vi "main.vi"() -> ()   [LabVIEW 2020]
uses:
  <vilib>/Platform/TimedLoop/XDataNode/wakeup.ctl
  <vilib>/Platform/TimedLoop/XDataNode/XDNodeRunTimeDep.lvlib
  <vilib>/Platform/TimedLoop/XDataNode/nitl_modes.ctl
  <vilib>/Platform/TimedLoop/XDataNode/timing_clust.ctl
  <vilib>/Platform/TimedLoop/XDataNode/XDataNode.xnode
  <vilib>/addons/control/pid/NI_PID_pid.lvlib
  <vilib>/addons/control/pid/pid.llb/PID (DBL).vi
  <vilib>/imathl/engines/lvmath/Functions/Error Handling/Create Error.vi
  <vilib>/imath/engines/lvmath2/RunTimeEngine/BuiltInFunctions/diag/NIMS_diag.vi
  <vilib>/imath/engines/lvmath2/RunTimeEngine/NodeEndStatement/NIMS_NodeEndStatement_Output.vi
  <vilib>/imath/engines/lvmath2/RunTimeEngine/ErrorHandling/NIMS_Finalize Error.vi
  <vilib>/imath/engines/lvmath2/RunTimeEngine/IndexReplace/NIMS M($,S)=V.vi
  <vilib>/imath/engines/lvmath2/RunTimeEngine/IndexRead/NIMS V(S).vi
  <vilib>/imath/engines/lvmath2/RunTimeEngine/ErrorHandling/NIMS_Create Error From Enums.vi
  <vilib>/imath/engines/lvmath2/RunTimeEngine/RangeToken/NIMS_Range_R2 - Integer.vi
  <vilib>/imath/engines/lvmath2/RunTimeEngine/VariableToken/NIMS_VariableToken_CondDefinedDefinedByReplace.vi
  <vilib>/imath/engines/lvmath2/RunTimeEngine/IndexReplace/NIMS V(S)=S.vi
  <vilib>/imath/engines/lvmath2/RunTimeEngine/CommandStatement/MC_CommandStatement_break.vi
  <vilib>/imath/engines/lvmath2/RunTimeEngine/VariableToken/NIMS_VariableToken_CondDefined.vi
  <vilib>/imath/engines/lvmath2/RunTimeEngine/IndexRead/NIMS V($).vi
  <vilib>/imath/engines/lvmath2/RunTimeEngine/ArithmeticOperatorToken/NIMS_ArithmeticOperator_rightdiv(C,C).vi
  <vilib>/imath/engines/lvmath2/RunTimeEngine/ArithmeticOperatorToken/NIMS_ArithmeticOperator_minus.vi
  <vilib>/imath/engines/lvmath2/RunTimeEngine/ArithmeticOperatorToken/NIMS_ArithmeticOperator_times.vi
  <vilib>/imath/engines/lvmath2/RunTimeEngine/ArithmeticOperatorToken/NIMS_ArithmeticOperator_plus.vi
  <vilib>/imath/engines/lvmath2/RunTimeEngine/ArithmeticOperatorToken/NIMS_ArithmeticOperator_multmx(M,CV).vi
  <vilib>/imath/engines/lvmath2/RunTimeEngine/ArithmeticOperatorToken/NIMS_ArithmeticOperator_multmx(M,CV)-internal.vi
  <vilib>/imath/engines/lvmath2/RunTimeEngine/ArithmeticOperatorToken/NIMS_ArithmeticOperator_multmx.vi
  <vilib>/imath/engines/lvmath2/RunTimeEngine/ArithmeticOperatorToken/NIMS_ArithmeticOperator_rightdiv.vi
  <vilib>/imath/engines/lvmath2/RunTimeEngine/MatrixToken/NIMS_MatrixToken_SorCV_M.vi
  <vilib>/imath/engines/lvmath2/RunTimeEngine/IndexRead/NIMS V(R2).vi
  <vilib>/imath/engines/lvmath2/RunTimeEngine/BuiltInFunctions/reshapemx/NIMS_[GM]_reshapemx.vi
  <vilib>/imath/engines/lvmath2/RunTimeEngine/IndexRead/NIMS M(S,$).vi
  <vilib>/imath/engines/lvmath2/RunTimeEngine/ArithmeticOperatorToken/NIMS_ArithmeticOperator_multmx(RV,CV).vi
  <vilib>/imath/engines/lvmath2/RunTimeEngine/IndexReplace/NIMS V(S)=M.vi
  <vilib>/imath/engines/lvmath2/RunTimeEngine/IndexRead/NIMS M(S).vi
  <vilib>/imath/engines/lvmath2/RunTimeEngine/ArithmeticOperatorToken/NIMS_ArithmeticOperator_rightdivmx(C,C).vi
  <vilib>/imath/engines/lvmath2/RunTimeEngine/BuiltInFunctions/max/2 inputs/NIMS_max(CG,CG)-no size check.vi
  <vilib>/imath/engines/lvmath2/RunTimeEngine/BuiltInFunctions/min/2 inputs/NIMS_min(CG,CG)-no size check.vi
  <vilib>/imath/engines/lvmath2/RunTimeEngine/IndexReplace/NIMS M(S)=S.vi
  <vilib>/imath/engines/lvmath2/RunTimeEngine/NodeEndStatement/NIMS_NodeEndStatement_Get Vector.vi
  <vilib>/imath/engines/lvmath2/RunTimeEngine/NodeEndStatement/NIMS_NodeEndStatement_Get Scalar.vi
  <vilib>/imath/engines/lvmath/Functions/Error Handling/MergeErrorsWrapper.vi
panel:
  out "e2":dbl[](array[numeric])
  out "e3":dbl[](array[numeric])
  out "e2_e3":dbl[](array[numeric])
  in  "选项卡控件":enum32{"液压机械臂操作面板", "软体操作面板 2"}(tab)
  out "No error controller":bool
  out "No error":bool
  in  "pin3":dbl(slide)=-87.9816513761468 scale=-160.0..-53.0
  in  "pin2":dbl(slide)=33.853211009174316 scale=-20.0..90.0
  in  "Swing 2":T1={"Open P2P Traj"=TRUE, "Open Sine Traj"=FALSE, "Open Ramp Traj"=FALSE, "Open DIY Traj"=FALSE} caption="Swing"
  in  "Boom 2":T1={"Open P2P Traj"=TRUE, "Open Sine Traj"=FALSE, "Open Ramp Traj"=FALSE, "Open DIY Traj"=FALSE} caption="Boom"
  in  "Stick 2":T1={"Open P2P Traj"=TRUE, "Open Sine Traj"=FALSE, "Open Ramp Traj"=FALSE, "Open DIY Traj"=FALSE} caption="Stick"
  in  "pin1":dbl(slide)=40.50458715596331 scale=-60.0..55.0
  in  "v_max_Stick":dbl=-20.0
  in  "a_max_Stick":dbl=-20.0
  in  "p_end_Stick":dbl=-40.0
  in  "t-whole_Stick":i32=300
  in  "v_max Boom":dbl=-20.0
  in  "a_max Boom":dbl=-20.0
  in  "p_end Boom":dbl=-40.0
  in  "t-whole_Boom":i32=300
  in  "v_max Swing":dbl=-20.0
  in  "a_max Swing":dbl=-20.0
  in  "p_end Swing":dbl=-40.0
  in  "t-whole_Swing":i32=300
  in  "bias Stick":dbl=60.0
  in  "bias Boom":dbl=-80.0
  in  "bias Swing":dbl
  in  "OpenLoop":T2={"Swing"=TRUE, "Boom"=TRUE, "Stick"=TRUE, "Swing_U"=-1.0, "Boom_U"=1.0, "Stick_U"=-1.0}
  out "?":bool
  out "?":bool
  in  "PID gains 3":T3={"proportional gain (Kc)"=0.15, "integral time (Ti, min)"=0.003, "derivative time (Td, min)"=1e-05} caption="PID增益" {"derivative time (Td, min)" step=0.001 format="%.6f"; "integral time (Ti, min)" step=0.001 format="%.6f"; "proportional gain (Kc)" step=0.01 format="%.6f"}
  in  "PID gains 2":T3={"proportional gain (Kc)"=0.15, "integral time (Ti, min)"=0.003, "derivative time (Td, min)"=0.0005} caption="PID增益" {"derivative time (Td, min)" format="%.6f"; "integral time (Ti, min)" format="%.6f"; "proportional gain (Kc)" format="%.6f"}
  out "?":bool
  in  "PID gains":T3={"proportional gain (Kc)"=0.15, "integral time (Ti, min)"=0.003, "derivative time (Td, min)"=0.0005} caption="PID增益" {"derivative time (Td, min)" format="%.6f"; "integral time (Ti, min)" format="%.6f"; "proportional gain (Kc)" step=0.01 format="%.6f"}
  out "minus":dbl format="%#_10g"
  out "real time(s)":dbl
  out "millisecond timer value":u32
  out "Angle_Swing":dbl
  out "Angle_Boom":dbl
  out "Angle_Stick":dbl
  in  "CloseLoop":T4 caption="ARC开关"
  out "?":string="Now OpenLoop is running"
  out "?":string="Now OpenLoop is running"
  out "?":string="Now OpenLoop is running"
  in  "K1":dbl[](array[numeric])=[80.0, 80.0, 80.0]
  in  "K2":dbl[](array[numeric])=[650.0, 850.0, 800.0]
  in  "K3(E-8)":dbl[](array[numeric])=[0.8, 1.0, 4.0] format="%#_8g"
  in  "Stickj？(F)":bool=TRUE
  in  "Boom？(F)":bool=TRUE
  in  "Swing？(F)":bool=TRUE
  in  "STOP/Return to save position":bool=TRUE
  in  "sw_QLda1":bool=TRUE
  in  "sw_FLda1":bool=TRUE
  in  "gamma_d1":dbl[](array[numeric])=[250.0, 6000.1, 6000.1]
  in  "gamma_d2(E-8)":dbl[](array[numeric])=[6.5, 3.1, 5.0]
  in  "sw_d1hat":bool
  in  "sw_d2hat":bool
  in  "w1":dbl[](array[numeric])=[0.26, 1.1, 0.07]
  in  "w2":dbl[](array[numeric])=[1414.0, 4000.0, 3020.0]
  in  "sw_Y_Q":bool
  in  "Save Data":bool
  in  "保存路径":path=path "C:/Qmz/data1.bin"
  in  "Stop\nTheta_Update":bool=TRUE
  in  "Use\nPreset_Theta":bool
  in  "Theta_s1_init":dbl[](array[numeric])=[500.0, 66.0, 30.0, 53.0, 57.0, 31.0, -10.0, -73.0, 77.0]
  in  "Theta_s2_init(E-8)":dbl[](array[numeric])=[2.0, 2.3, 2.5, 0.0, 100.0, 10.0, 0.0, -99.0, -200.0]
  out "ARC_U":dbl[](array[numeric])
  in  "Cluster":T5={"valve1Switch"=FALSE, "valve2Switch"=FALSE, "valve3Switch"=FALSE, "valve4Switch"=TRUE, "valve5Switch"=FALSE, "valve6Switch"=TRUE} caption="簇"
  in  "开始控制 2":bool
  in  "reinitialize? (F)":bool=TRUE caption="重新初始化？(F)"
  in  "PID gains 4":T3={"proportional gain (Kc)"=43.0, "integral time (Ti, min)"=0.1, "derivative time (Td, min)"=0.0001} caption="PID增益" {"derivative time (Td, min)" format="%.6f"; "integral time (Ti, min)" format="%.7f"; "proportional gain (Kc)" format="%.3f"}
  out "Pressure":T6(graph)
  out "理想弯曲角":dbl(graph)=20.0
  out "PID输出":dbl(graph)=570.8164856437539
  out "实际弯曲角":dbl(graph)=6.725198008284792
  in  "手动输入":dbl
  in  "启用自动输入":bool
  out "速度输入":dbl
  out "误差":dbl(graph)=13.274801991715208
  out "Theta_Boom_F_hat_next":T7(graph)
  out "Theta_Boom_Q_hat_next":T7(graph)
  out "Theta_Stick_Q_hat_next":T7(graph)
  out "Theta_Stick_F_hat_next":T7(graph)
  out "F_Boom":cluster{dbl, dbl, dbl, dbl}(graph)
  out "Q_Swing":cluster{dbl, dbl, dbl, dbl}(graph)
  out "Q_Boom":cluster{dbl, dbl, dbl, dbl}(graph)
  out "F_Stick":cluster{dbl, dbl, dbl, dbl}(graph)
  out "Q_Stick":cluster{dbl, dbl, dbl, dbl}(graph)
  out "F_Swing":cluster{dbl, dbl, dbl, dbl}(graph)
  out "Esti_e2":T8(graph)={"FLda1[0]"=125.504748463915, "FLda1[1]"=53.955555282260676, "FLda1[2]"=-93.06627669799211}
  out "Esti_e1":T8(graph)={"FLda1[0]"=125.504748463915, "FLda1[1]"=53.955555282260676, "FLda1[2]"=-93.06627669799211}
  out "Swing":T9(graph)
  out "Stick":T9(graph)
  out "Boom":T9(graph)
  out "Theta_Boom_Q_hat_next":dbl[](array[numeric])
  out "Theta_Boom_F_hat_next":dbl[](array[numeric])
  out "Theta_Swing_Q_hat_next":dbl[](array[numeric])
  out "Theta_Swing_F_hat_next":dbl[](array[numeric])
  out "Theta_Stick_Q_hat_next":dbl[](array[numeric])
  out "Theta_Stick_F_hat_next":dbl[](array[numeric])
  # "上到下\n*Ld \\ *Lda1 \\ *Lds2 \\ *Lda2"
  # "fv"
  # "fc"
  # "D_n"
  # "D_Q2"
  # "D_Q1"
  # "1/beta"
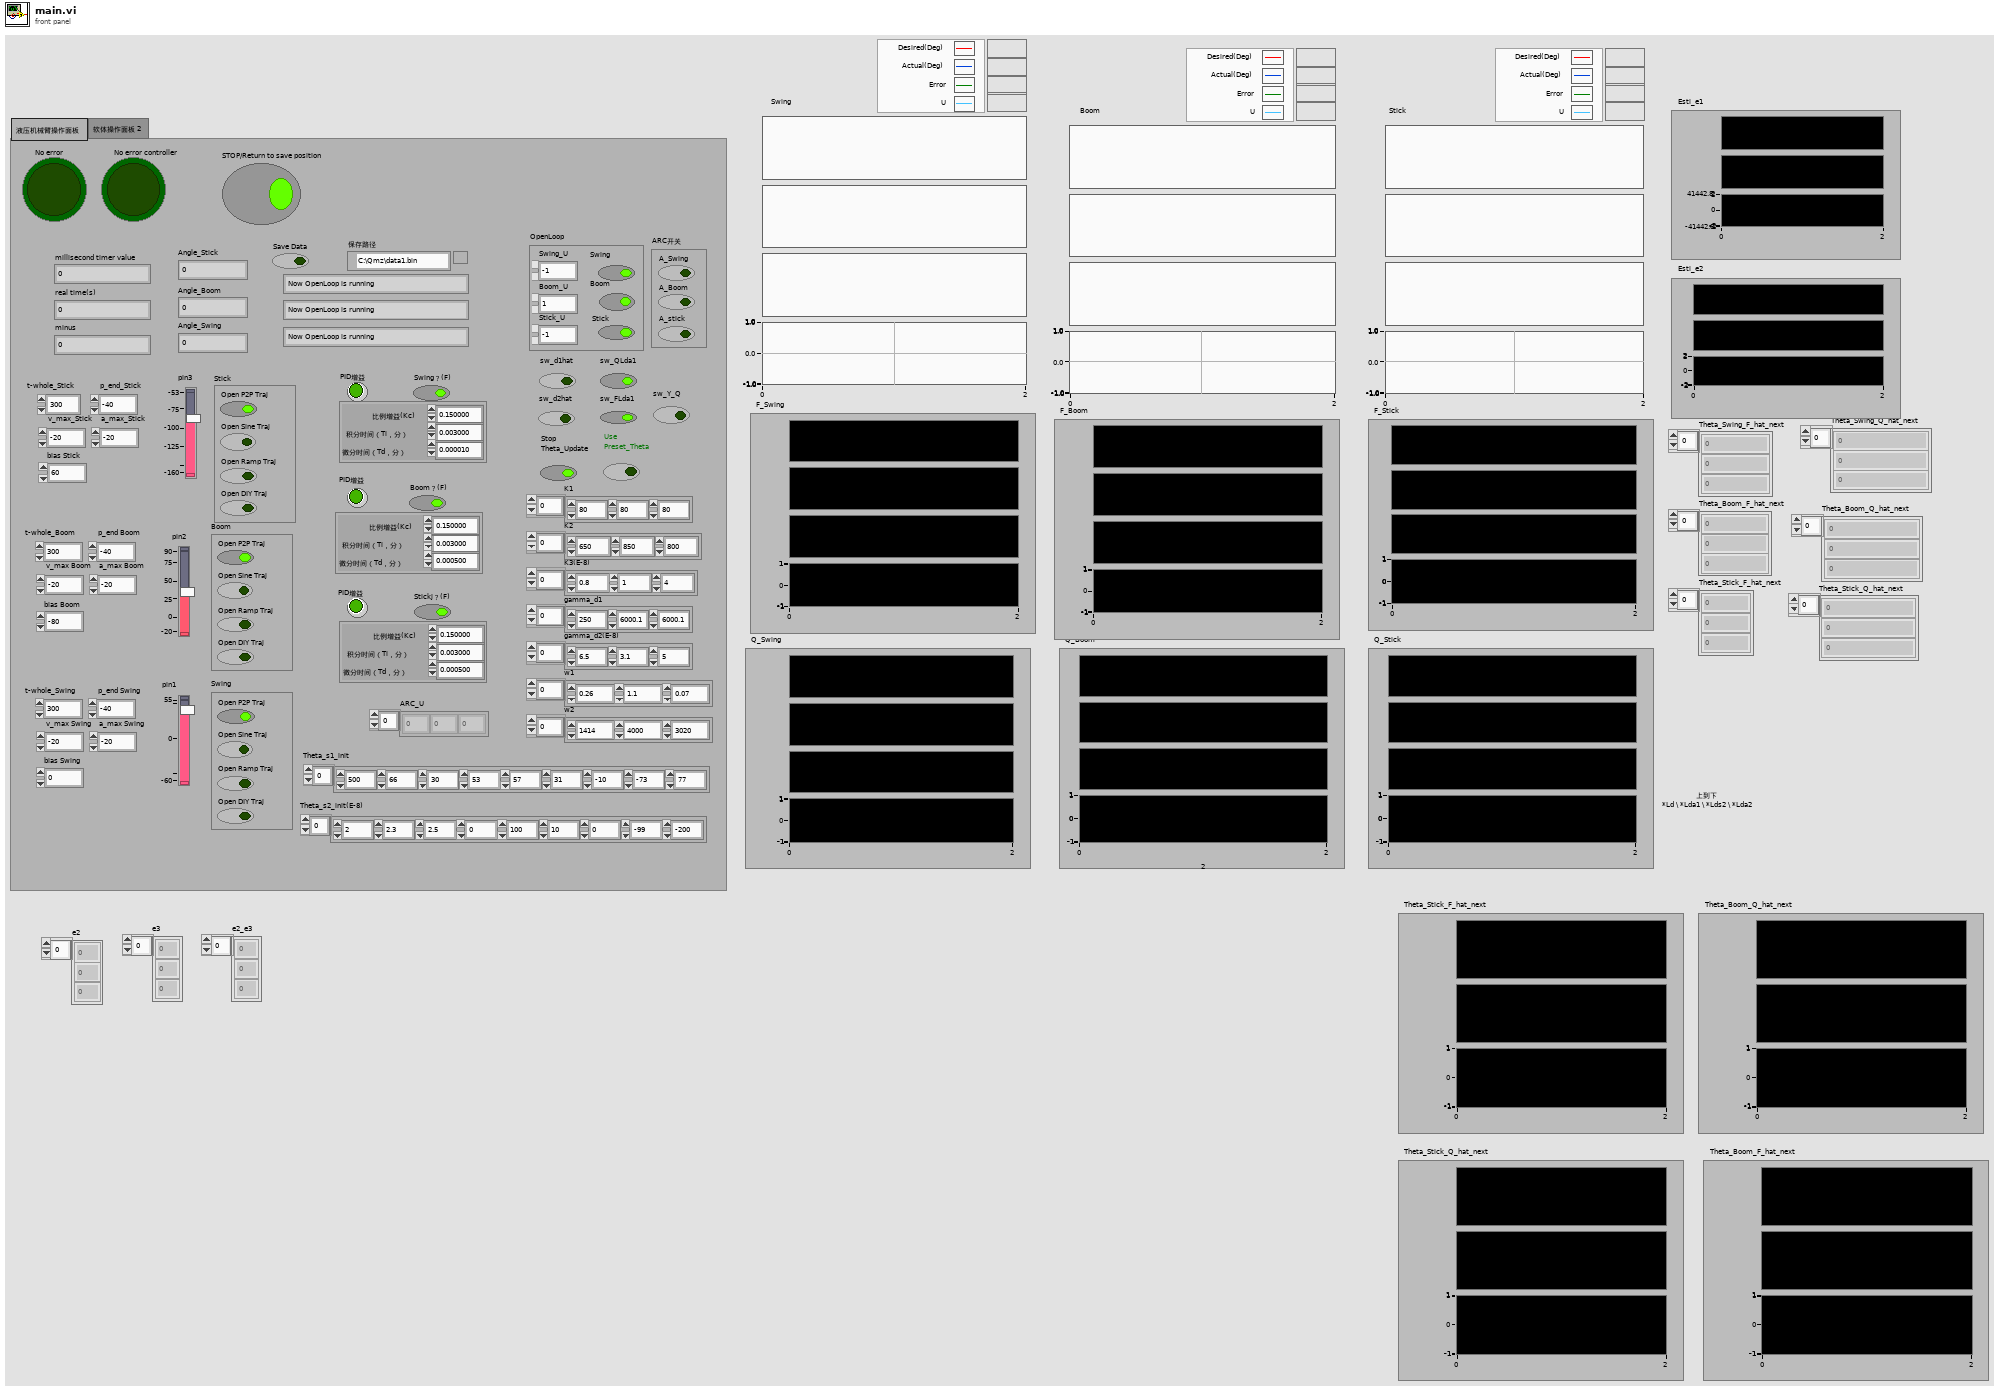
[diagram p1: front panel]
types:
  T1 = cluster{"Open P2P Traj":bool, "Open Sine Traj":bool, "Open Ramp Traj":bool, "Open DIY Traj":bool}
  T2 = cluster{"Swing":bool, "Boom":bool, "Stick":bool, "Swing_U":dbl, "Boom_U":dbl, "Stick_U":dbl}
  T3 = cluster{"proportional gain (Kc)":dbl, "integral time (Ti, min)":dbl, "derivative time (Td, min)":dbl}
  T4 = cluster{"A_Swing":bool, "A_Boom":bool, "A_stick\n":bool}
  T5 = cluster{"valve1Switch":bool, "valve2Switch":bool, "valve3Switch":bool, "valve4Switch":bool, "valve5Switch":bool, "valve6Switch":bool}
  T6 = cluster{"Double":dbl, "Double":dbl, "Double":dbl}
  T7 = cluster{"Theta_Stick_F_hat_next[0]":dbl, "Theta_Stick_F_hat_next[1]":dbl, "Theta_Stick_F_hat_next[2]":dbl}
  T8 = cluster{"FLda1[0]":dbl, "FLda1[1]":dbl, "FLda1[2]":dbl}
  T9 = cluster{"Double":dbl, "Double":dbl, "Double":dbl, "Double":dbl}
  T10 = typedef "XDNodeRunTimeDep.lvlib/timing_clust.ctl" = cluster{"Expected End [f-1]":u64, "Actual End [f-1]":u64, "Finished Late? [f-1]":bool, "Expected End [i-1]":u64, "Actual End [i-1]":u64, "Finished Late? [i-1]":bool, "Expected Start [i]":u64, "Actual Start [i]":u64, "Expected Start [f]":u64, "Actual Start [f]":u64, "Source Name":string, "Structure Name":string, "Period":i64, "Deadline":i64, "Offset":i64, "Start":i64, "Priority":i32, "Timeout":i32, "Mode":T11, "Wakeup Reason":T12, "Error":errorcluster, "Source Type":string, "Secondary Source Type":string, "Global End Time":u64, "Global Start Time":u64, "Frame Duration":u64, "Iteration Duration":u64, "Assigned CPU":i32, "I/O Scan Engine Mode":u32}
  T11 = typedef "XDNodeRunTimeDep.lvlib/nitl_modes.ctl" = enum32{"No Change", "Process missed periods, maintain original phase", "Discard missed periods, maintain original phase", "Process missed periods, ignore original phase", "Discard missed periods, ignore original phase"}
  T12 = typedef "XDNodeRunTimeDep.lvlib/wakeup.ctl" = enum32{"Normal", "Aborted", "Asynchronous wakeup", "Timing source error", "Timed loop error", "Timeout"}
  T13 = cluster{"Q_Stick[0]":cdb, "Q_Stick[1]":cdb, "Q_Stick[2]":cdb, "Q_Stick[3]":cdb}
  T14 = cluster{"Q_Boom[0]":cdb, "Q_Boom[1]":cdb, "Q_Boom[2]":cdb, "Q_Boom[3]":cdb}
  T15 = cluster{"Q_Swing[0]":cdb, "Q_Swing[1]":cdb, "Q_Swing[2]":cdb, "Q_Swing[3]":cdb}
  T16 = cluster{"F_Stick[0]":cdb, "F_Stick[1]":cdb, "F_Stick[2]":cdb, "F_Stick[3]":cdb}
  T17 = cluster{"F_Boom[0]":cdb, "F_Boom[1]":cdb, "F_Boom[2]":cdb, "F_Boom[3]":cdb}
  T18 = cluster{"F_Swing[0]":cdb, "F_Swing[1]":cdb, "F_Swing[2]":cdb, "F_Swing[3]":cdb}
  T19 = cluster{"Epsilon_1[0]":cdb, "Epsilon_1[1]":cdb, "Epsilon_1[2]":cdb}
  T20 = cluster{"Epsilon_2[0]":cdb, "Epsilon_2[1]":cdb, "Epsilon_2[2]":cdb}
  T21 = cluster{"Theta_Stick_Q_hat_next[0]":dbl, "Theta_Stick_Q_hat_next[1]":dbl, "Theta_Stick_Q_hat_next[2]":dbl}
  T22 = cluster{"Theta_Boom_Q_hat_next[0]":dbl, "Theta_Boom_Q_hat_next[1]":dbl, "Theta_Boom_Q_hat_next[2]":dbl}
  T23 = cluster{"Theta_Boom_F_hat_next[0]":dbl, "Theta_Boom_F_hat_next[1]":dbl, "Theta_Boom_F_hat_next[2]":dbl}
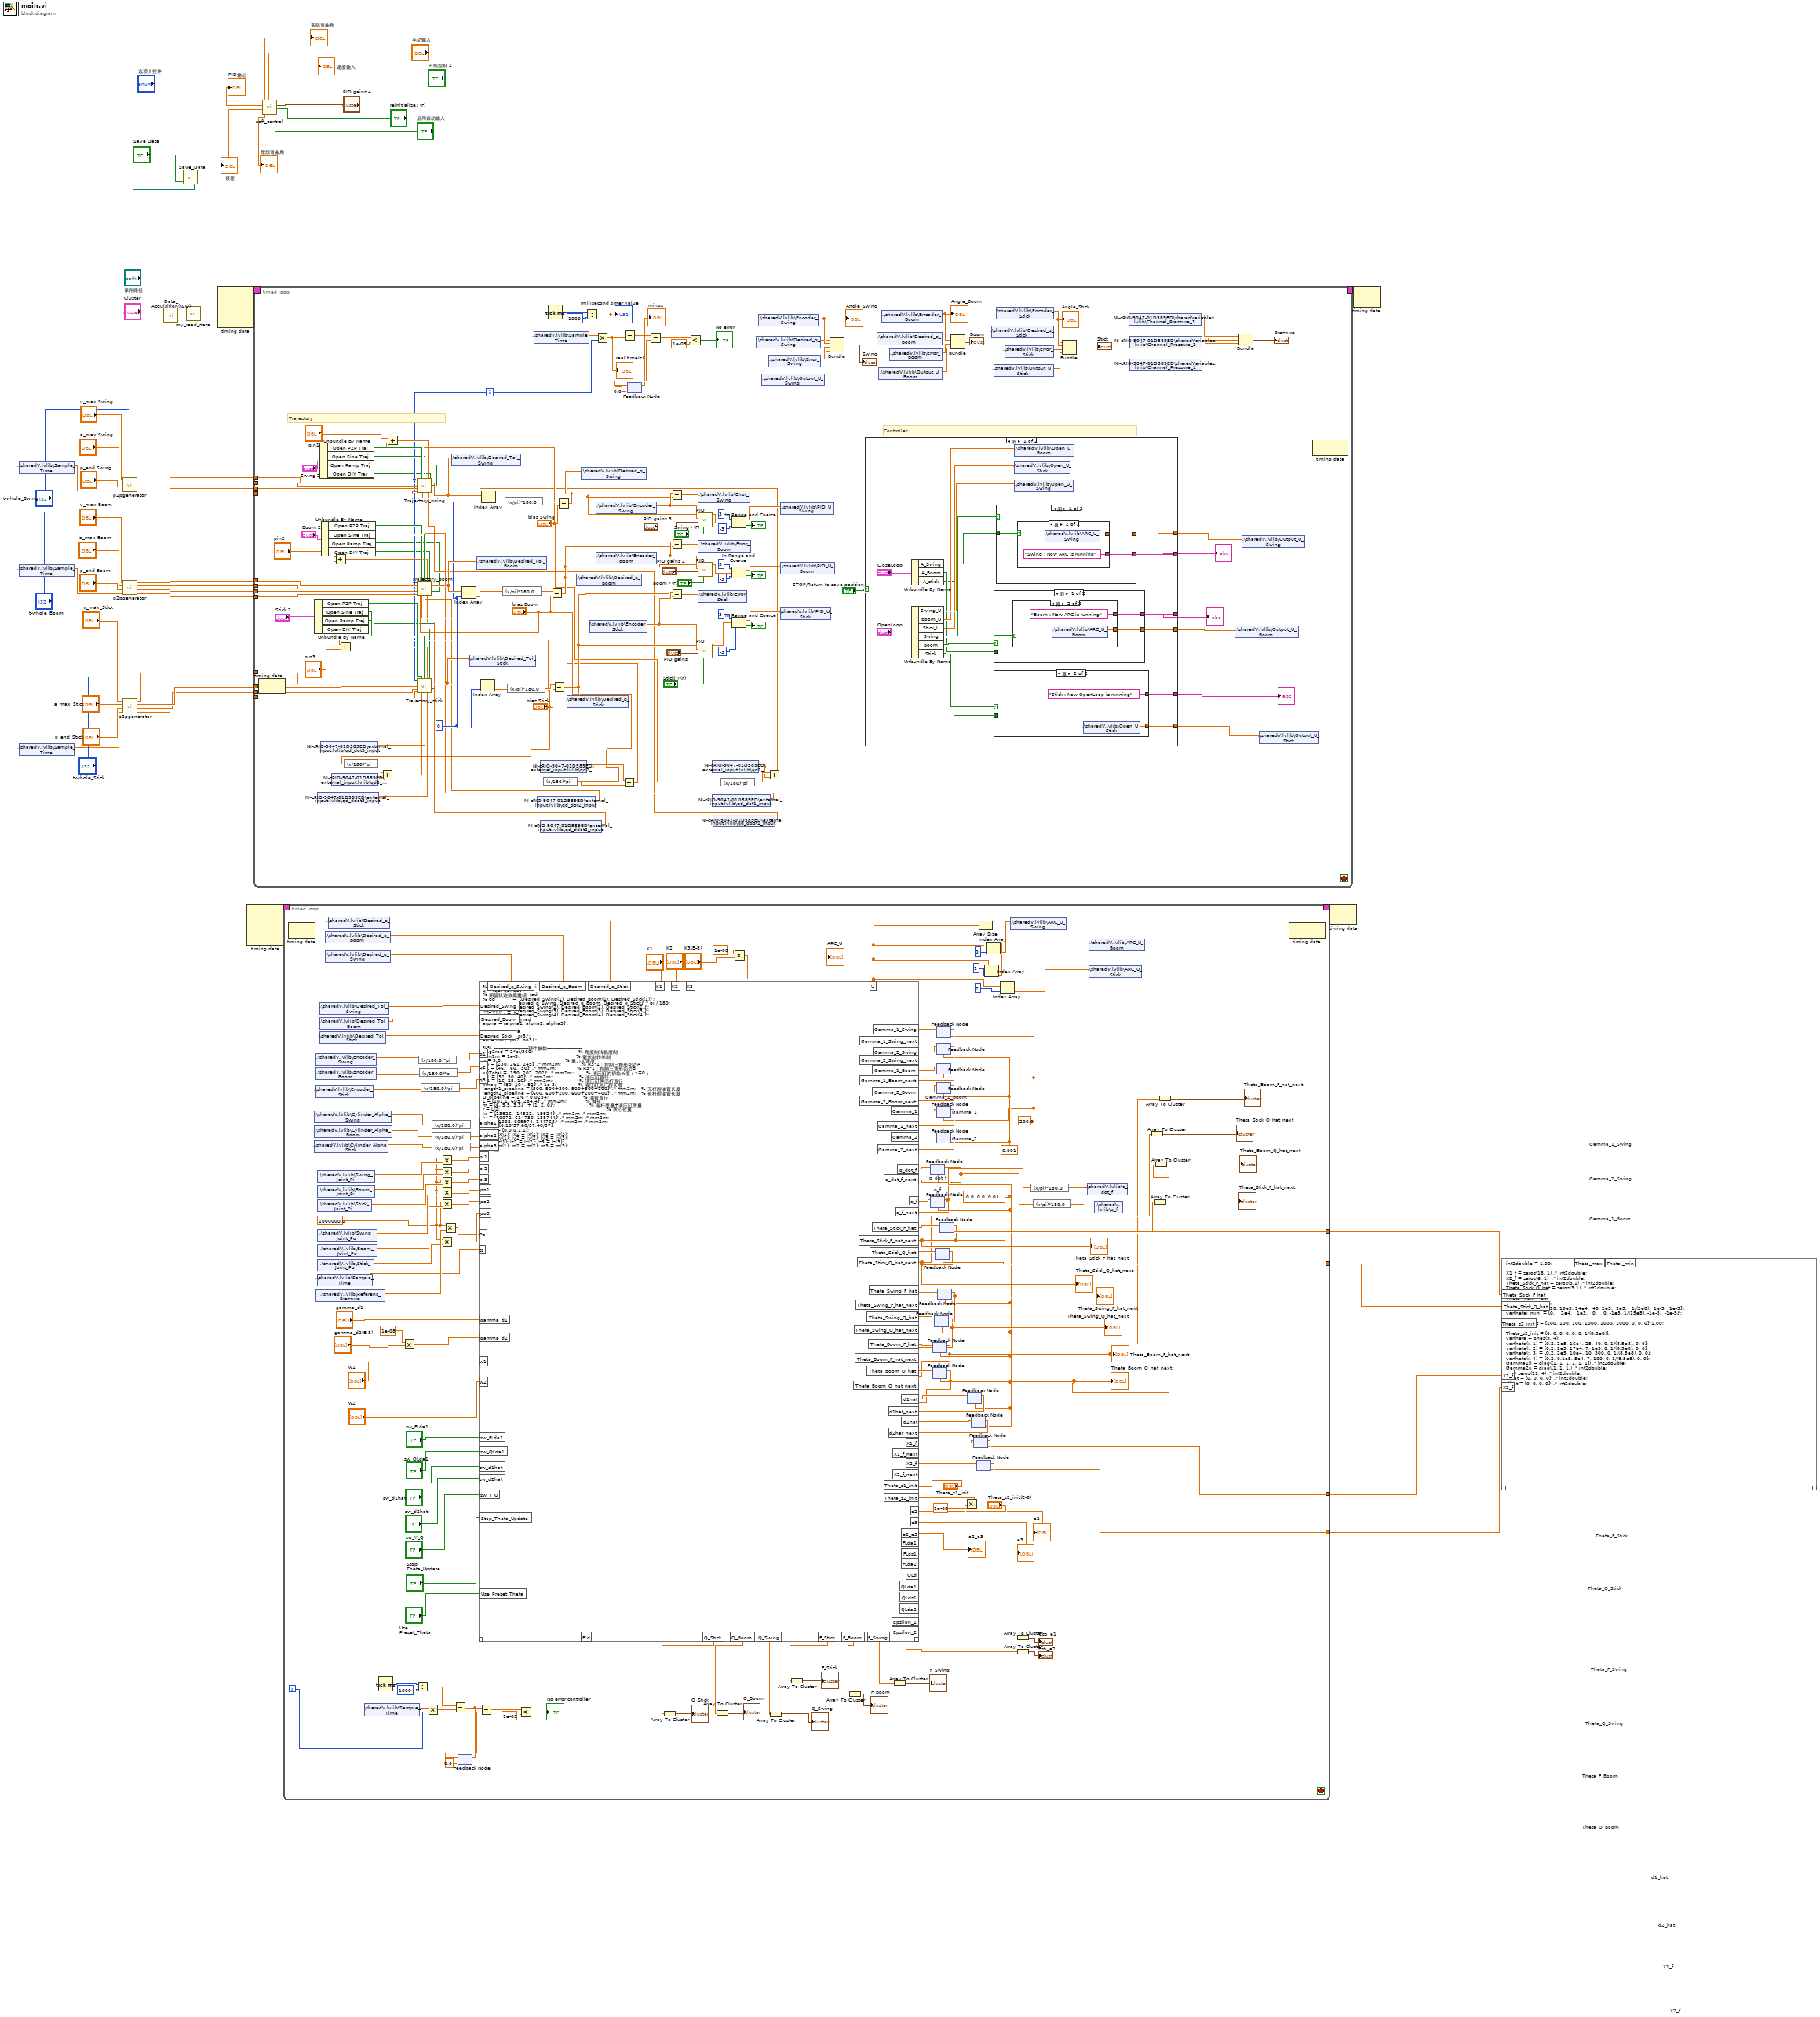
[diagram p0: block diagram]
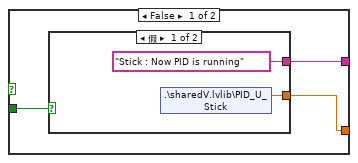
[diagram p2: hidden frame]
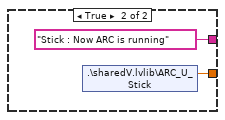
[diagram p3: hidden frame]
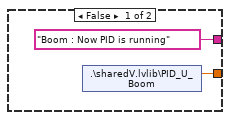
[diagram p4: hidden frame]
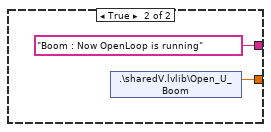
[diagram p5: hidden frame]
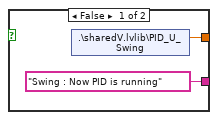
[diagram p6: hidden frame]
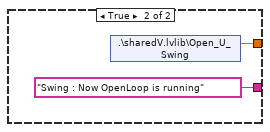
[diagram p7: hidden frame]
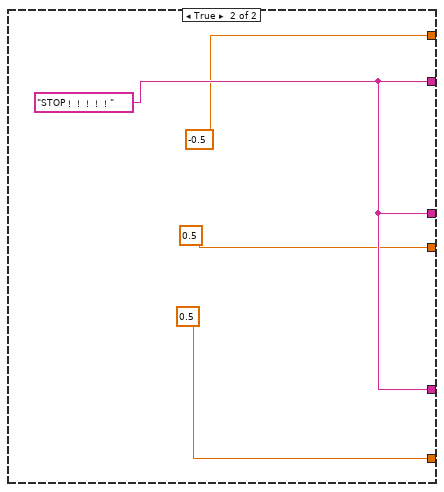
[diagram p8: hidden frame]
diagram:
  n1 = shared-variable ".\\sharedV.lvlib\\Sample_Time"() -> (w29:dbl)  [unwired: 1 in, 1 out]
  n2 = shared-variable ".\\sharedV.lvlib\\Sample_Time"() -> (w34:dbl)  [unwired: 1 in, 1 out]
  n3 = shared-variable ".\\sharedV.lvlib\\Sample_Time"() -> (w14:dbl)  [unwired: 1 in, 1 out]
  n4 = call "p2pgenerator.vi"("whole time for p2p"="t-whole_Swing", "ts"=w29, "p_end"="p_end Swing", "a_max"="a_max Swing", "v_max"="v_max Swing") -> ("jerk"=w21:dbl[], "a"=w22:dbl[], "v"=w23:dbl[], "s"=w24:dbl[])  [unwired: 3 in]
  n5 = call "p2pgenerator.vi"("whole time for p2p"="t-whole_Boom", "ts"=w34, "p_end"="p_end Boom", "a_max"="a_max Boom", "v_max"="v_max Boom") -> ("jerk"=w25:dbl[], "a"=w26:dbl[], "v"=w27:dbl[], "s"=w28:dbl[])  [unwired: 3 in]
  n6 = call "p2pgenerator.vi"("whole time for p2p"="t-whole_Stick", "ts"=w14, "p_end"="p_end_Stick", "a_max"="a_max_Stick", "v_max"="v_max_Stick") -> ("jerk"=w39:dbl[], "a"=w40:dbl[], "v"=w41:dbl[], "s"=w42:dbl[])  [unwired: 3 in]
  n7 = call "Data_Acquisition(I&O).vi"("Cluster"="Cluster") -> ()  [unwired: 11 in]
  n8 = call "Save_Data.vi"("保存路径"="保存路径", "Save Data"="Save Data") -> ()  [unwired: 4 in]
  n9 = call "my_read_data.vi"() -> ()  [unwired: 12 in]
  n10 = node-c288() -> (w48:T10)  [unwired: 4 in]
  n11 = node-c288() -> (w20:T10)  [unwired: 4 in]
  n12 = timed-loop {
    timing: w48 -> [_]
    timing-out: [_] -> w47
    tunnel: w42 -> [w174]
    tunnel: w41 -> [w177]
    tunnel: w40 -> [w176]
    tunnel: w39 -> [w175]
    tunnel: w28 -> [w173]
    tunnel: w27 -> [w172]
    tunnel: w26 -> [w171]
    tunnel: w25 -> [w170]
    tunnel: w24 -> [w160]
    tunnel: w23 -> [w159]
    tunnel: w22 -> [w158]
    tunnel: w21 -> [w157]
    i -> [w59]
    stop <- _ stop-if-true
    w131 = 0
    # "Controller"
    # "Trajectory"
    n13 = node-c288() -> ()  [unwired: 1 in, 1 out]
    n14 = Unbundle By Name("Stick 2") -> ("Open P2P Traj"=w168:bool, "Open Sine Traj"=w167:bool, "Open Ramp Traj"=w53:bool, "Open DIY Traj"=w54:bool)
    n15 = shared-variable "NI-cRIO-9047-01D589ED\\external_input.lvlib\\qd_ddot3_input"() -> (w101:dbl[])  [unwired: 1 in, 1 out]
    n16 = Unbundle By Name("Swing 2") -> ("Open P2P Traj"=w164:bool, "Open Sine Traj"=w163:bool, "Open Ramp Traj"=w49:bool, "Open DIY Traj"=w50:bool)
    n17 = shared-variable "NI-cRIO-9047-01D589ED\\external_input.lvlib\\qd_dot3_input"() -> (w100:dbl[])  [unwired: 1 in, 1 out]
    n18 = Unbundle By Name("Boom 2") -> ("Open P2P Traj"=w161:bool, "Open Sine Traj"=w162:bool, "Open Ramp Traj"=w52:bool, "Open DIY Traj"=w51:bool)
    n19 = shared-variable "NI-cRIO-9047-01D589ED\\external_input.lvlib\\qd3_input"() -> (w99:dbl[])  [unwired: 1 in, 1 out]
    n20 = Add(x="pin2", y="bias Boom") -> (x+y=w107:dbl)
    n21 = Add(x="bias Stick", y="pin3") -> (x+y=w108:dbl)
    n22 = expression code="(x/180)*pi" ("弧度转换至角度")("bias Stick") -> (w102:dbl)
    n23 = Add(x=w102, y=w99) -> (x+y=w98:dbl[])
    n24 = Add(x="pin1", y="bias Swing") -> (x+y=w104:dbl)
    n25 = call "Trajectory_stick.vi"("i"=w59, "if p2p"=w168, "ifSin?"=w167, "Target_Angle"=w108, "if_DIY"=w54, "q"=w174, "qd"=w177, "qdd"=w176, "if_Ramp"=w53, "qddd"=w175, "qd8_1"=w98, "qd8_dot_2"=w100, "qd8_ddot_2"=w101) -> ("qd1_tol"=w110:dbl[])  [unwired: 2 in]
    n26 = shared-variable ".\\sharedV.lvlib\\Desired_Tol_Stick"(w110) -> ()  [unwired: 1 in, 1 out]
    n27 = Index Array(array=w110, index=w131) -> (element=w128:dbl)
    n28 = expression code="(x/pi)*180.0" ("弧度转换至角度")(w128) -> (w127:dbl)
    n29 = shared-variable ".\\sharedV.lvlib\\Sample_Time"() -> (w60:dbl)  [unwired: 1 in, 1 out]
    n30 = shared-variable "NI-cRIO-9047-01D589ED\\external_input.lvlib\\qd_dot2_input"() -> (w93:dbl[])  [unwired: 1 in, 1 out]
    n31 = shared-variable "NI-cRIO-9047-01D589ED\\external_input.lvlib\\qd2_input"() -> (w97:dbl[])  [unwired: 1 in, 1 out]
    n32 = shared-variable "NI-cRIO-9047-01D589ED\\external_input.lvlib\\qd_ddot2_input"() -> (w92:dbl[])  [unwired: 1 in, 1 out]
    n33 = expression code="(x/180)*pi" ("弧度转换至角度")("bias Boom") -> (w95:dbl)
    n34 = Tick Count (ms)() -> (millisecond timer value=w62:u32)
    n35 = Subtract(x=w127, y="bias Stick") -> (x-y=w121:dbl)
    n36 = shared-variable ".\\sharedV.lvlib\\Desired_q_Stick"(w121) -> ()  [unwired: 1 in, 1 out]
    n37 = Divide(x=w62, y=u32 1000) -> (x/y=w64:dbl)
    "millisecond timer value" <- w64
    n38 = shared-variable ".\\sharedV.lvlib\\Encoder_Stick"() -> (w122:dbl)  [unwired: 1 in, 1 out]
    n39 = Multiply(x=w60, y=w59) -> (x*y=w61:dbl)
    "real time(s)" <- w61
    n40 = shared-variable ".\\sharedV.lvlib\\Encoder_Swing"() -> (w118:dbl)  [unwired: 1 in, 1 out]
    n41 = shared-variable ".\\sharedV.lvlib\\Encoder_Boom"() -> (w120:dbl)  [unwired: 1 in, 1 out]
    n42 = Add(x=w97, y=w95) -> (x+y=w94:dbl[])
    n43 = call "Trajectory_boom.vi"("i"=w59, "if p2p"=w161, "ifSin?"=w162, "Target_Angle"=w107, "if end8"=w51, "q"=w173, "qd"=w172, "qdd"=w171, "if  Ramp"=w52, "qddd"=w170, "qd8_1"=w94, "qd8_dot_2"=w93, "qd8_ddot_2"=w92) -> ("qd1_tol"=w135:dbl[])  [unwired: 2 in]
    n44 = Index Array(array=w135, index=w131) -> (element=w134:dbl)
    n45 = shared-variable ".\\sharedV.lvlib\\Desired_Tol_Boom"(w135) -> ()  [unwired: 1 in, 1 out]
    n46 = expression code="(x/pi)*180.0" ("弧度转换至角度")(w134) -> (w156:dbl)
    n47 = Subtract(x=w156, y="bias Boom") -> (x-y=w119:dbl)
    n48 = shared-variable ".\\sharedV.lvlib\\Desired_q_Boom"(w119) -> ()  [unwired: 1 in, 1 out]
    n49 = Subtract(x=w64, y=w61) -> (x-y=w68:dbl)
    "minus" <- w68
    n50 = feedback #1(0.0) -> (w69:dbl)
    n51 = feedback-in #1(w68) -> ()
    n52 = Subtract(x=w68, y=w69) -> (x-y=w65:dbl)
    n53 = Subtract(x=w120, y=w119) -> (x-y=w133:dbl)
    n54 = Subtract(x=w122, y=w121) -> (x-y=w115:dbl)
    n55 = Less?(x=w65, y=1e-05) -> (x < y?=→"No error":bool)
    n56 = shared-variable ".\\sharedV.lvlib\\Error_Boom"(w133) -> ()  [unwired: 1 in, 1 out]
    n57 = call-poly <vilib>:"PID.vi"("reinitialize? (F)"="Boom？(F)", "PID gains"="PID gains 2", "process variable"=w120, "setpoint"=w119) -> ("output"=w149:dbl)  [unwired: 6 in, 1 out]
    n58 = shared-variable ".\\sharedV.lvlib\\Error_Stick"(w115) -> ()  [unwired: 1 in, 1 out]
    n59 = call-poly <vilib>:"PID.vi"("reinitialize? (F)"="Stickj？(F)", "PID gains"="PID gains", "process variable"=w122, "setpoint"=w121) -> ("output"=w126:dbl)  [unwired: 6 in, 1 out]
    n60 = shared-variable "NI-cRIO-9047-01D589ED\\external_input.lvlib\\qd1_input"() -> (w89:dbl[])  [unwired: 1 in, 1 out]
    n61 = shared-variable "NI-cRIO-9047-01D589ED\\external_input.lvlib\\qd_dot1_input"() -> (w87:dbl[])  [unwired: 1 in, 1 out]
    n62 = shared-variable "NI-cRIO-9047-01D589ED\\external_input.lvlib\\qd_ddot1_input"() -> (w86:dbl[])  [unwired: 1 in, 1 out]
    n63 = expression code="(x/180)*pi" ("弧度转换至角度")("bias Swing") -> (w90:dbl)
    n64 = In Range and Coerce(upper limit=3, x=w149, lower limit=-3) -> (coerced(x)=w140:dbl, In Range?=→"?":bool)
    n65 = In Range and Coerce(upper limit=3, x=w126, lower limit=-3) -> (coerced(x)=w141:dbl, In Range?=→"?":bool)
    n66 = shared-variable ".\\sharedV.lvlib\\Desired_q_Swing"() -> (w71:dbl)  [unwired: 1 in, 1 out]
    n67 = shared-variable ".\\sharedV.lvlib\\Encoder_Swing"() -> (w79:dbl)  [unwired: 1 in, 1 out]
    "Angle_Swing" <- w79
    n68 = shared-variable ".\\sharedV.lvlib\\Output_U_Swing"() -> (w73:dbl)  [unwired: 1 in, 1 out]
    n69 = Add(x=w90, y=w89) -> (x+y=w88:dbl[])
    n70 = call "Trajectory_swing.vi"("i"=w59, "if p2p"=w164, "ifSin?"=w163, "Target_Angle"=w104, "if end8"=w50, "q"=w160, "qd"=w159, "if Ramp"=w49, "qdd"=w158, "qddd"=w157, "qd8_1"=w88, "qd8_dot_2"=w87, "qd8_ddot_2"=w86) -> ("qd1_tol"=w132:dbl[])  [unwired: 2 in]
    n71 = shared-variable ".\\sharedV.lvlib\\Desired_Tol_Swing"(w132) -> ()  [unwired: 1 in, 1 out]
    n72 = Index Array(array=w132, index=w131) -> (element=w130:dbl)
    n73 = expression code="(x/pi)*180.0" ("弧度转换至角度")(w130) -> (w111:dbl)
    n74 = Subtract(x=w111, y="bias Swing") -> (x-y=w117:dbl)
    n75 = shared-variable ".\\sharedV.lvlib\\Desired_q_Swing"(w117) -> ()  [unwired: 1 in, 1 out]
    n76 = Subtract(x=w118, y=w117) -> (x-y=w129:dbl)
    n77 = shared-variable ".\\sharedV.lvlib\\Error_Swing"(w129) -> ()  [unwired: 1 in, 1 out]
    n78 = call-poly <vilib>:"PID.vi"("reinitialize? (F)"="Swing？(F)", "PID gains"="PID gains 3", "process variable"=w118, "setpoint"=w117) -> ("output"=w155:dbl)  [unwired: 6 in, 1 out]
    n79 = In Range and Coerce(upper limit=3, x=w155, lower limit=-3) -> (coerced(x)=w139:dbl, In Range?=→"?":bool)
    n80 = shared-variable ".\\sharedV.lvlib\\Error_Swing"() -> (w72:dbl)  [unwired: 1 in, 1 out]
    n81 = shared-variable ".\\sharedV.lvlib\\PID_U_Swing"(w139) -> ()  [unwired: 1 in, 1 out]
    n82 = shared-variable ".\\sharedV.lvlib\\PID_U_Boom"(w140) -> ()  [unwired: 1 in, 1 out]
    n83 = shared-variable ".\\sharedV.lvlib\\PID_U_Stick"(w141) -> ()  [unwired: 1 in, 1 out]
    n84 = Bundle("Double"=w71, "Double"=w79, "Double"=w72, "Double"=w73) -> (→"Swing":T9)  [unwired: 1 in]
    n85 = case shown="假" "STOP/Return to save position" {
      tunnel: [w188 -0.5] -> w114
      tunnel: [w186 w225] -> w138
      tunnel: [w183 w225] -> w137
      tunnel: [w182 0.5] -> w113
      tunnel: [w181 w225] -> w136
      tunnel: [w180 0.5] -> w112
      frame False {
        n86 = Unbundle By Name("CloseLoop") -> ("A_Swing"=w187:bool, "A_Boom"=w184:bool, "A_stick"=w178:bool)
        n87 = Unbundle By Name("OpenLoop") -> ("Swing_U"=w193:dbl, "Boom_U"=w191:dbl, "Stick_U"=w190:dbl, "Swing"=w189:bool, "Boom"=w185:bool, "Stick"=w179:bool)
        n88 = case shown="假" w185 {
          tunnel: [w204 w212] -> w182
          tunnel: w184 -> [w206 _]
          tunnel: [w205 "Boom : Now OpenLoop is running"] -> w183
          frame False {
            n89 = case shown="真" w206 {
              tunnel: ["Boom : Now PID is running" "Boom : Now ARC is running"] -> w205
              tunnel: [w207 w209] -> w204
              frame False {
                n90 = shared-variable ".\\sharedV.lvlib\\PID_U_Boom"() -> (w207:dbl)  [unwired: 1 in, 1 out]
              }
              frame True {
                n91 = shared-variable ".\\sharedV.lvlib\\ARC_U_Boom"() -> (w209:dbl)  [unwired: 1 in, 1 out]
              }
            }
          }
          frame True {
            n92 = shared-variable ".\\sharedV.lvlib\\Open_U_Boom"() -> (w212:dbl)  [unwired: 1 in, 1 out]
          }
        }
        n93 = case shown="真" w179 {
          tunnel: [w195 w203] -> w180
          tunnel: w178 -> [w197 _]
          tunnel: [w196 "Stick : Now OpenLoop is running"] -> w181
          frame False {
            n94 = case shown="假" w197 {
              tunnel: ["Stick : Now PID is running" "Stick : Now ARC is running"] -> w196
              tunnel: [w198 w200] -> w195
              frame False {
                n95 = shared-variable ".\\sharedV.lvlib\\PID_U_Stick"() -> (w198:dbl)  [unwired: 1 in, 1 out]
              }
              frame True {
                n96 = shared-variable ".\\sharedV.lvlib\\ARC_U_Stick"() -> (w200:dbl)  [unwired: 1 in, 1 out]
              }
            }
          }
          frame True {
            n97 = shared-variable ".\\sharedV.lvlib\\Open_U_Stick"() -> (w203:dbl)  [unwired: 1 in, 1 out]
          }
        }
        n98 = case shown="假" w189 {
          tunnel: [w213 w221] -> w188
          tunnel: w187 -> [w215 _]
          tunnel: [w214 "Swing : Now OpenLoop is running"] -> w186
          frame False {
            n99 = case shown="真" w215 {
              tunnel: ["Swing : Now PID is running" "Swing : Now ARC is running"] -> w214
              tunnel: [w216 w218] -> w213
              frame False {
                n100 = shared-variable ".\\sharedV.lvlib\\PID_U_Swing"() -> (w216:dbl)  [unwired: 1 in, 1 out]
              }
              frame True {
                n101 = shared-variable ".\\sharedV.lvlib\\ARC_U_Swing"() -> (w218:dbl)  [unwired: 1 in, 1 out]
              }
            }
          }
          frame True {
            n102 = shared-variable ".\\sharedV.lvlib\\Open_U_Swing"() -> (w221:dbl)  [unwired: 1 in, 1 out]
          }
        }
        n103 = shared-variable ".\\sharedV.lvlib\\Open_U_Boom"(w191) -> ()  [unwired: 1 in, 1 out]
        n104 = shared-variable ".\\sharedV.lvlib\\Open_U_Stick"(w190) -> ()  [unwired: 1 in, 1 out]
        n105 = shared-variable ".\\sharedV.lvlib\\Open_U_Swing"(w193) -> ()  [unwired: 1 in, 1 out]
      }
      frame True {
        w225 = "STOP！！！！！"
      }
    }
    "?" <- w138
    "?" <- w137
    "?" <- w136
    n106 = shared-variable ".\\sharedV.lvlib\\Desired_q_Boom"() -> (w75:dbl)  [unwired: 1 in, 1 out]
    n107 = shared-variable ".\\sharedV.lvlib\\Output_U_Boom"() -> (w78:dbl)  [unwired: 1 in, 1 out]
    n108 = shared-variable ".\\sharedV.lvlib\\Encoder_Boom"() -> (w76:dbl)  [unwired: 1 in, 1 out]
    "Angle_Boom" <- w76
    n109 = shared-variable ".\\sharedV.lvlib\\Error_Boom"() -> (w77:dbl)  [unwired: 1 in, 1 out]
    n110 = Bundle("Double"=w75, "Double"=w76, "Double"=w77, "Double"=w78) -> (→"Boom":T9)  [unwired: 1 in]
    n111 = shared-variable ".\\sharedV.lvlib\\Desired_q_Stick"() -> (w82:dbl)  [unwired: 1 in, 1 out]
    n112 = shared-variable ".\\sharedV.lvlib\\Output_U_Stick"() -> (w80:dbl)  [unwired: 1 in, 1 out]
    n113 = shared-variable ".\\sharedV.lvlib\\Encoder_Stick"() -> (w83:dbl)  [unwired: 1 in, 1 out]
    "Angle_Stick" <- w83
    n114 = shared-variable ".\\sharedV.lvlib\\Error_Stick"() -> (w81:dbl)  [unwired: 1 in, 1 out]
    n115 = Bundle("Double"=w82, "Double"=w83, "Double"=w81, "Double"=w80) -> (→"Stick":T9)  [unwired: 1 in]
    n116 = shared-variable "NI-cRIO-9047-01D589ED\\sharedVariables.lvlib\\Channel_Pressure_3"() -> (w57:dbl)  [unwired: 1 in, 1 out]
    n117 = shared-variable "NI-cRIO-9047-01D589ED\\sharedVariables.lvlib\\Channel_Pressure_2"() -> (w56:dbl)  [unwired: 1 in, 1 out]
    n118 = shared-variable "NI-cRIO-9047-01D589ED\\sharedVariables.lvlib\\Channel_Pressure_1"() -> (w55:dbl)  [unwired: 1 in, 1 out]
    n119 = shared-variable ".\\sharedV.lvlib\\Output_U_Boom"(w113) -> ()  [unwired: 1 in, 1 out]
    n120 = Bundle("Double"=w57, "Double"=w56, "Double"=w55) -> (→"Pressure":T6)  [unwired: 1 in]
    n121 = shared-variable ".\\sharedV.lvlib\\Output_U_Swing"(w114) -> ()  [unwired: 1 in, 1 out]
    n122 = shared-variable ".\\sharedV.lvlib\\Output_U_Stick"(w112) -> ()  [unwired: 1 in, 1 out]
    n123 = node-c288() -> ()  [unwired: 1 in, 1 out]
  }
  n124 = call "soft_control.vi"("手动输入"="手动输入", "开始控制"="开始控制 2", "PID gains"="PID gains 4", "reinitialize? (F)"="reinitialize? (F)", "启用自动输入"="启用自动输入") -> ("实际弯曲角"=→"实际弯曲角":dbl, "PID输出"=→"PID输出":dbl, "误差"=→"误差":dbl, "理想弯曲角"=→"理想弯曲角":dbl, "速度输入"=→"速度输入":dbl)  [unwired: 1 in]
  n125 = node-c288(w47) -> ()  [unwired: 1 out]
  n126 = mathscript code="int2double = 1.00;\n\nX1_f = zeros(18, 1) .* int2double;\nX2_f = zeros(6, 1)  .* int2double;\nTheta_Stick_F_hat = zeros(3,1) .* int2double;\nTheta_Stick_Q_hat = zeros(3,1) .* int2double;\n\nTheta_max = 20;\nThetai_min  = -20;\nvarthetai_max = [20, 10e5, 24e4,  48, 2e3,  1e5,   1/(2e8),  1e-5,  1e-5]';\nvarthetai_min  = [0,    2e4,   1e3,   0,    0, -1e5, 1/(15e8), -1e-5,  -1e-5]';\n\nTheta_s1_init = [100, 100, 100, 1000, 1000, 1000, 0, 0, 0]*1.00;\n\nTheta_s2_init = [0, 0, 0, 0, 0, 0, 1/(8.5e8)];\nvartheta = ones(9, 4);\nvartheta(:, 1) = [0.2, 2e5, 16e4, 25, 40, 0, 1/(8.5e8), 0, 0];\nvartheta(:, 2) = [0.2, 2e5, 17e4, 7, 1e3, 0, 1/(8.5e8), 0, 0];\nvartheta(:, 3) = [0.2, 2e5, 10e4, 10, 300, 0, 1/(8.5e8), 0, 0];\nvartheta(:, 4) = [0.2, 0.1e5, 5e4, 7, 100, 0, 1/(8.5e8), 0, 0];\nGamma1ii = diag([1, 1, 1, 1, 1, 1]) .* int2double;\nGamma2ii = diag([1, 1, 1]) .* int2double;\nXf = zeros(11, 4) .* int2double;\ndihat = [0, 0, 0, 0]' .* int2double;\nzihat = [0, 0, 0, 0]' .* int2double;"() -> ("Theta_Stick_F_hat"=w16:dbl[], "X1_f"=w18:dbl[], "X2_f"=w17:dbl[], "Theta_Stick_Q_hat"=w15:dbl[])  [unwired: 1 in, 4 out]
  n127 = timed-loop {
    timing: w20 -> [_]
    timing-out: [_] -> w19
    tunnel: w18 -> [w306]
    tunnel: w17 -> [w305]
    tunnel: w16 -> [w303]
    tunnel: w15 -> [w301]
    i -> [w229]
    stop <- _ stop-if-true
    w256 = 0.001
    w255 = 200.0
    w271 = dbl[] [0.0, 0.0, 0.0]
    w348 = 1000000.0
    n128 = node-c288() -> ()  [unwired: 1 in, 1 out]
    n129 = shared-variable ".\\sharedV.lvlib\\Cylinder_Alpha_Swing"() -> (w369:dbl)  [unwired: 1 in, 1 out]
    n130 = shared-variable ".\\sharedV.lvlib\\Cylinder_Alpha_Boom"() -> (w366:dbl)  [unwired: 1 in, 1 out]
    n131 = shared-variable ".\\sharedV.lvlib\\Cylinder_Alpha_Stick"() -> (w365:dbl)  [unwired: 1 in, 1 out]
    n132 = shared-variable ".\\sharedV.lvlib\\Encoder_Swing"() -> (w347:dbl)  [unwired: 1 in, 1 out]
    n133 = shared-variable ".\\sharedV.lvlib\\Encoder_Boom"() -> (w346:dbl)  [unwired: 1 in, 1 out]
    n134 = shared-variable ".\\sharedV.lvlib\\Encoder_Stick"() -> (w345:dbl)  [unwired: 1 in, 1 out]
    n135 = shared-variable ".\\sharedV.lvlib\\Referenc_Pressure"() -> (w351:dbl)  [unwired: 1 in, 1 out]
    n136 = shared-variable ".\\sharedV.lvlib\\Swing_Joint_Pi"() -> (w363:dbl)  [unwired: 1 in, 1 out]
    n137 = shared-variable ".\\sharedV.lvlib\\Boom_Joint_Pi"() -> (w361:dbl)  [unwired: 1 in, 1 out]
    n138 = shared-variable ".\\sharedV.lvlib\\Stick_Joint_Pi"() -> (w360:dbl)  [unwired: 1 in, 1 out]
    n139 = shared-variable ".\\sharedV.lvlib\\Swing_Joint_Po"() -> (w359:dbl)  [unwired: 1 in, 1 out]
    n140 = shared-variable ".\\sharedV.lvlib\\Boom_Joint_Po"() -> (w358:dbl)  [unwired: 1 in, 1 out]
    n141 = shared-variable ".\\sharedV.lvlib\\Stick_Joint_Po"() -> (w343:dbl)  [unwired: 1 in, 1 out]
    n142 = shared-variable ".\\sharedV.lvlib\\Sample_Time"() -> (w344:dbl)  [unwired: 1 in, 1 out]
    n143 = shared-variable ".\\sharedV.lvlib\\Desired_Tol_Swing"() -> (w335:dbl[])  [unwired: 1 in, 1 out]
    n144 = shared-variable ".\\sharedV.lvlib\\Desired_Tol_Boom"() -> (w334:dbl[])  [unwired: 1 in, 1 out]
    n145 = shared-variable ".\\sharedV.lvlib\\Desired_Tol_Stick"() -> (w333:dbl[])  [unwired: 1 in, 1 out]
    n146 = shared-variable ".\\sharedV.lvlib\\Desired_q_Boom"() -> (w327:dbl)  [unwired: 1 in, 1 out]
    n147 = shared-variable ".\\sharedV.lvlib\\Desired_q_Swing"() -> (w326:dbl)  [unwired: 1 in, 1 out]
    n148 = shared-variable ".\\sharedV.lvlib\\Desired_q_Stick"() -> (w328:dbl)  [unwired: 1 in, 1 out]
    n149 = shared-variable ".\\sharedV.lvlib\\Sample_Time"() -> (w239:dbl)  [unwired: 1 in, 1 out]
    n150 = Tick Count (ms)() -> (millisecond timer value=w228:u32)
    n151 = Multiply(x=1e-08, y="gamma_d2(E-8)") -> (x*y=w321:dbl[])
    n152 = Divide(x=w228, y=u32 1000) -> (x/y=w236:dbl)
    n153 = expression code="(x/180.0)*pi"(w347) -> (w370:dbl)
    n154 = expression code="(x/180.0)*pi"(w346) -> (w332:dbl)
    n155 = expression code="(x/180.0)*pi"(w345) -> (w331:dbl)
    n156 = Multiply(x=w239, y=w229) -> (x*y=w238:dbl)
    n157 = expression code="(x/180.0)*pi"(w369) -> (w368:dbl)
    n158 = expression code="(x/180.0)*pi"(w366) -> (w367:dbl)
    n159 = expression code="(x/180.0)*pi"(w365) -> (w364:dbl)
    n160 = Multiply(x=w348, y=w363) -> (x*y=w362:dbl)
    n161 = Multiply(x=w348, y=w361) -> (x*y=w353:dbl)
    n162 = Multiply(x=w348, y=w360) -> (x*y=w354:dbl)
    n163 = Multiply(x=w348, y=w359) -> (x*y=w355:dbl)
    n164 = Multiply(x=w348, y=w358) -> (x*y=w356:dbl)
    n165 = Multiply(x=w348, y=w343) -> (x*y=w357:dbl)
    n166 = Multiply(x=w348, y=w351) -> (x*y=w352:dbl)
    n167 = Subtract(x=w236, y=w238) -> (x-y=w232:dbl)
    n168 = feedback #2(0.0) -> (w231:dbl)
    n169 = feedback-in #2(w232) -> ()
    n170 = Subtract(x=w232, y=w231) -> (x-y=w235:dbl)
    n171 = Less?(x=w235, y=1e-05) -> (x < y?=→"No error controller":bool)
    n172 = Multiply ("乘")(x=1e-08, y="K3(E-8)") -> (x*y=w318:dbl[])
    n173 = feedback #3 "q_dot_f"(w271) -> (w272:dbl[])
    n174 = feedback #4 "q_f"(w271) -> (w273:dbl[])
    n175 = feedback #5 "Theta_F_Boom"(w271) -> (w296:dbl[])
    n176 = feedback #6 "Theta_Q_Boom"(w271) -> (w295:dbl[])
    n177 = feedback #7 "Theta_Q_Swing"(w271) -> (w298:dbl[])
    n178 = feedback #8 "Theta_Q_Stick"(w301) -> (w302:dbl[])
    n179 = feedback #9 "Gamma_1_Swing"(w255) -> (w268:dbl)
    n180 = feedback #10 "Gamma_2_Swing"(w256) -> (w266:dbl)
    n181 = feedback #11 "Gamma_1_Boom"(w255) -> (w264:dbl)
    n182 = feedback #12 "Gamma_2_Boom"(w256) -> (w262:dbl)
    n183 = feedback #13 "Gamma_1"(w255) -> (w260:dbl)
    n184 = feedback #14 "Gamma_2"(w256) -> (w258:dbl)
    n185 = feedback #15 "Theta_F_Swing"(w271) -> (w300:dbl[])
    n186 = feedback #16 "Theta_F_Stick"(w303) -> (w304:dbl[])
    n187 = Multiply(x=1e-08, y="Theta_s2_init(E-8)") -> (x*y=w311:dbl[])
    n188 = feedback #17 "d1_hat"(w271) -> (w317:dbl[])
    n189 = feedback #18 "d2_hat"(w271) -> (w315:dbl[])
    n190 = feedback #19 "X1_f"(w306) -> (w310:dbl[])
    n191 = feedback #20 "X2_f"(w305) -> (w309:dbl[])
    n192 = mathscript code="%%Author : Manzhi Qi\nq = [q1, q2, q3]';\n% 期望轨迹数据重组  rad\n% qd           =  [Desired_Swing(1), Desired_Boom(1), Desired_Stick(1)]';\nqd           =  [Desired_q_Swing, Desired_q_Boom, Desired_q_Stick]' * pi / 180;\nqd_dot     =  [Desired_Swing(2), Desired_Boom(2), Desired_Stick(2)]';\nqd_ddot   =  [Desired_Swing(3), Desired_Boom(3), Desired_Stick(3)]';\nqd_dddot =  [Desired_Swing(4), Desired_Boom(4), Desired_Stick(4)]';\n% 控制三角形夹角 rad\nalpha = [alpha1, alpha2, alpha3]'; \n\n% 液压缸压力 Pa\nPi = [pi1, pi2, pi3]';\nPo = [po1, po2, po3]';\n\n%% ----------------------硬件参数----------------------\ndeg2rad = 2*pi/360;                             % 角度制转弧度制\nmm2m = 1e-3;                                    % 毫米制转米制\ng = 9.8;                                        % 重力加速度\nAB = [230, 261, 245]' .* mm2m;             % R3*1：控制三角形邻边A\nBC = [46,   60,  50]' .* mm2m;             % R3*1：控制三角形邻边B\nx0Total = [190, 207, 202]' .* mm2m;        % 液压缸的初始长度（x=0）\nD1 = [32, 50, 40]' .* mm2m;                 % 液压缸直径\nD2 = [16, 25, 16]' .* mm2m;                 % 液压缸伸出杆直径\nxmax = [80, 104, 82]' .* 1e-3;              % 液压缸总行程长度\nlength1_pipeline = [500, 500+300, 500+300+100]' .* mm2m;   % 无杆腔油管长度\nlength2_pipeline = [600, 600+200, 600+200+400]' .* mm2m;   % 有杆腔油管长度\nD_pipeline = 1/6 * 0.0254;                      % 油管直径\nL = [101.1, 605, 284.4]' .* mm2m;            % 臂长\nm = [6, 5.5, 3.3]'  + [1, 2, 0]';                      % 连杆质量+液压缸质量\nr = L/2;                                                                    % 质心位置\nIx = [13826,  14322,  19924]' .* mm2m .* mm2m;                        \nIy = [30072, 614730, 138744]' .* mm2m .* mm2m;                       \nIz = [21003, 609974, 144768]' .* mm2m .* mm2m;                       \n% q = [0,10/57,60/57,40/57];                                                \n% qd = [0,0,0.1,1];                                                      \nIx1 = Ix(1); Ix2 = Ix(2); Ix3 = Ix(3);\nIy1 = Iy(1); Iy2 = Iy(2); Iy3 = Iy(3);\nIz1 = Iz(1); Iz2 = Iz(2); Iz3 = Iz(3);\nm1 = m(1); m2 = m(2); m3 = m(3); \nr1 = r(1); r2 = r(2); r3 = r(3); \nL1 = L(1); L2 = L(2); L3 = L(3); \n\nfor ii = 1:3\n  xNowTotal(ii) = sqrt(AB(ii)^2 + BC(ii)^2 - 2*AB(ii)*BC(ii)*cos(alpha(ii)));           \t%控制三角形中关节角对应边长\nend\nxNowTotal = xNowTotal(:);\nJ_h = diag((AB .* BC .* sin(alpha)) ./ xNowTotal);\ninv_J_h = diag(xNowTotal./ (AB .* BC .* sin(alpha)));\n% 液压相关\nA_pipeline = 0.25*pi*D_pipeline^2;        \t        % 油管面积\nAi = 0.25*pi*D1.^2;                                 % 无杆腔面积\nAo = Ai - 0.25*pi*D2.^2;                      \t    % 有杆腔面积\nVh1 = A_pipeline .* length1_pipeline;               % 无杆腔油管油液体积\nVh2 = A_pipeline.*length2_pipeline + xmax.*Ao;      % 有杆腔油管油液体积\nxL = xNowTotal - x0Total;                           % 液压缸位移\nVi = Vh1 + Ai.*xL;                                  % 无杆腔油液总体积\nVo = Vh2 - Ao.*xL;                                  % 有杆腔油液总体积\nA_Q = Ai.^2./Vi + Ao.^2./Vo;\nB_Q = Ai ./ Vi;\nC_Q = Ao ./ Vo;\n\n% 二阶微分滤波求q_dot q_ddot.................\nq_dot_f = q_dot_f(:);\nq_f = q_f(:);\nq_dot = q_dot_f;\nwn = 100; % 原先是100，为了减少相位滞后，应当尽可能大\nepsilon = 0.707;\nq_ddot_f = wn^2*q - 2*epsilon*wn*q_dot_f - wn^2*q_f;\nq_dot_f_next = q_dot_f + q_ddot_f*ts;\nq_f_next = q_f + q_dot_f.*ts;\n\n%%\nq1d = q_dot(1);  q2d = q_dot(2);  q3d = q_dot(3); \nM =...\n[Ix2/2 + Ix3/2 + Iy2/2 + Iy3/2 + Iz1 - (Ix3*cos(2*q2 + 2*q3))/2 + (Iy3*cos(2*q2 + 2*q3))/2 + L1^2*m2 + L1^2*m3 + (L2^2*m3)/2 + (L3^2*m3)/2 + m1*r1^2 + (m2*r2^2)/2 - (Ix2*cos(2*q2))/2 + (Iy2*cos(2*q2))/2 + (L2^2*m3*cos(2*q2))/2 + (m2*r2^2*cos(2*q2))/2 + (L3^2*m3*cos(2*q2 + 2*q3))/2 + 2*L1*L3*m3*cos(q2 + q3) + 2*L1*L2*m3*cos(q2) + L2*L3*m3*cos(q3) + 2*L1*m2*r2*cos(q2) + L2*L3*m3*cos(2*q2 + q3),                                                            0,                                0;\n                                                                                                                                                                                                                                                                                                                                                                                                        0, m3*L2^2 + 2*m3*cos(q3)*L2*r3 + m2*r2^2 + m3*r3^2 + Iz2 + Iz3, m3*r3^2 + L2*m3*cos(q3)*r3 + Iz3;\n                                                                                                                                                                                                                                                                                                                                                                                                        0,                             m3*r3^2 + L2*m3*cos(q3)*r3 + Iz3,                    m3*r3^2 + Iz3];\n\nC =...\n[- q2d*((m3*sin(2*q2)*L2^2)/2 + m3*sin(2*q2 + q3)*L2*L3 + L1*m3*sin(q2)*L2 + (m3*sin(2*q2 + 2*q3)*L3^2)/2 + L1*m3*sin(q2 + q3)*L3 + (m2*sin(2*q2)*r2^2)/2 + L1*m2*sin(q2)*r2 - (Ix3*sin(2*q2 + 2*q3))/2 + (Iy3*sin(2*q2 + 2*q3))/2 - (Ix2*sin(2*q2))/2 + (Iy2*sin(2*q2))/2) - q3d*((Iy3*sin(2*q2 + 2*q3))/2 - (Ix3*sin(2*q2 + 2*q3))/2 + (L3^2*m3*sin(2*q2 + 2*q3))/2 + L1*L3*m3*sin(q2 + q3) + (L2*L3*m3*sin(q3))/2 + (L2*L3*m3*sin(2*q2 + q3))/2),  -q1d*((m3*sin(2*q2)*L2^2)/2 + m3*sin(2*q2 + q3)*L2*L3 + L1*m3*sin(q2)*L2 + (m3*sin(2*q2 + 2*q3)*L3^2)/2 + L1*m3*sin(q2 + q3)*L3 + (m2*sin(2*q2)*r2^2)/2 + L1*m2*sin(q2)*r2 - (Ix3*sin(2*q2 + 2*q3))/2 + (Iy3*sin(2*q2 + 2*q3))/2 - (Ix2*sin(2*q2))/2 + (Iy2*sin(2*q2))/2),  -q1d*((Iy3*sin(2*q2 + 2*q3))/2 - (Ix3*sin(2*q2 + 2*q3))/2 + (L3^2*m3*sin(2*q2 + 2*q3))/2 + L1*L3*m3*sin(q2 + q3) + (L2*L3*m3*sin(q3))/2 + (L2*L3*m3*sin(2*q2 + q3))/2);\n                                                                                                                                                                           q1d*((m3*sin(2*q2)*L2^2)/2 + m3*sin(2*q2 + q3)*L2*L3 + L1*m3*sin(q2)*L2 + (m3*sin(2*q2 + 2*q3)*L3^2)/2 + L1*m3*sin(q2 + q3)*L3 + (m2*sin(2*q2)*r2^2)/2 + L1*m2*sin(q2)*r2 - (Ix3*sin(2*q2 + 2*q3))/2 + (Iy3*sin(2*q2 + 2*q3))/2 - (Ix2*sin(2*q2))/2 + (Iy2*sin(2*q2))/2),                                                                                                                                                                                                                                                      -L2*m3*q3d*r3*sin(q3),                                                                                                                                           -L2*m3*r3*sin(q3)*(q2d + q3d);\n                                                                                                                                                                                                                                                                              q1d*((Iy3*sin(2*q2 + 2*q3))/2 - (Ix3*sin(2*q2 + 2*q3))/2 + (L3^2*m3*sin(2*q2 + 2*q3))/2 + L1*L3*m3*sin(q2 + q3) + (L2*L3*m3*sin(q3))/2 + (L2*L3*m3*sin(2*q2 + q3))/2),                                                                                                                                                                                                                                                       L2*m3*q2d*r3*sin(q3),                                                                                                                                                                       0;];\n\nG = [                                                    0;\n    g*(m2*r2*cos(q2) + m3*r3*cos(q2 + q3) + L2*m3*cos(q2));\n                                      g*m3*r3*cos(q2 + q3);] ;\n\n\nq1d_d = qd_dot(1);  q2d_d = qd_dot(2);  q3d_d = qd_dot(3); \nq1_d = qd(1);  q2_d = qd(2);  q3_d = qd(3); \nM_d =...\n[Ix2/2 + Ix3/2 + Iy2/2 + Iy3/2 + Iz1 - (Ix3*cos(2*q2_d + 2*q3_d))/2 + (Iy3*cos(2*q2_d + 2*q3_d))/2 + L1^2*m2 + L1^2*m3 + (L2^2*m3)/2 + (L3^2*m3)/2 + m1*r1^2 + (m2*r2^2)/2 - (Ix2*cos(2*q2_d))/2 + (Iy2*cos(2*q2_d))/2 + (L2^2*m3*cos(2*q2_d))/2 + (m2*r2^2*cos(2*q2_d))/2 + (L3^2*m3*cos(2*q2_d + 2*q3_d))/2 + 2*L1*L3*m3*cos(q2_d + q3_d) + 2*L1*L2*m3*cos(q2_d) + L2*L3*m3*cos(q3_d) + 2*L1*m2*r2*cos(q2_d) + L2*L3*m3*cos(2*q2_d + q3_d),                                                            0,                                0;\n                                                                                                                                                                                                                                                                                                                                                                                                        0, m3*L2^2 + 2*m3*cos(q3_d)*L2*r3 + m2*r2^2 + m3*r3^2 + Iz2 + Iz3, m3*r3^2 + L2*m3*cos(q3_d)*r3 + Iz3;\n                                                                                                                                                                                                                                                                                                                                                                                                        0,                             m3*r3^2 + L2*m3*cos(q3_d)*r3 + Iz3,                    m3*r3^2 + Iz3];\n\nC_d =...\n[- q2d_d*((m3*sin(2*q2_d)*L2^2)/2 + m3*sin(2*q2_d + q3_d)*L2*L3 + L1*m3*sin(q2_d)*L2 + (m3*sin(2*q2_d + 2*q3_d)*L3^2)/2 + L1*m3*sin(q2_d + q3_d)*L3 + (m2*sin(2*q2_d)*r2^2)/2 + L1*m2*sin(q2_d)*r2 - (Ix3*sin(2*q2_d + 2*q3_d))/2 + (Iy3*sin(2*q2_d + 2*q3_d))/2 - (Ix2*sin(2*q2_d))/2 + (Iy2*sin(2*q2_d))/2) - q3d_d*((Iy3*sin(2*q2_d + 2*q3_d))/2 - (Ix3*sin(2*q2_d + 2*q3_d))/2 + (L3^2*m3*sin(2*q2_d + 2*q3_d))/2 + L1*L3*m3*sin(q2_d + q3_d) + (L2*L3*m3*sin(q3_d))/2 + (L2*L3*m3*sin(2*q2_d + q3_d))/2),  -q1d_d*((m3*sin(2*q2_d)*L2^2)/2 + m3*sin(2*q2_d + q3_d)*L2*L3 + L1*m3*sin(q2_d)*L2 + (m3*sin(2*q2_d + 2*q3_d)*L3^2)/2 + L1*m3*sin(q2_d + q3_d)*L3 + (m2*sin(2*q2_d)*r2^2)/2 + L1*m2*sin(q2_d)*r2 - (Ix3*sin(2*q2_d + 2*q3_d))/2 + (Iy3*sin(2*q2_d + 2*q3_d))/2 - (Ix2*sin(2*q2_d))/2 + (Iy2*sin(2*q2_d))/2),  -q1d_d*((Iy3*sin(2*q2_d + 2*q3_d))/2 - (Ix3*sin(2*q2_d + 2*q3_d))/2 + (L3^2*m3*sin(2*q2_d + 2*q3_d))/2 + L1*L3*m3*sin(q2_d + q3_d) + (L2*L3*m3*sin(q3_d))/2 + (L2*L3*m3*sin(2*q2_d + q3_d))/2);\n                                                                                                                                                                           q1d_d*((m3*sin(2*q2_d)*L2^2)/2 + m3*sin(2*q2_d + q3_d)*L2*L3 + L1*m3*sin(q2_d)*L2 + (m3*sin(2*q2_d + 2*q3_d)*L3^2)/2 + L1*m3*sin(q2_d + q3_d)*L3 + (m2*sin(2*q2_d)*r2^2)/2 + L1*m2*sin(q2_d)*r2 - (Ix3*sin(2*q2_d + 2*q3_d))/2 + (Iy3*sin(2*q2_d + 2*q3_d))/2 - (Ix2*sin(2*q2_d))/2 + (Iy2*sin(2*q2_d))/2),                                                                                                                                                                                                                                                      -L2*m3*q3d_d*r3*sin(q3_d),                                                                                                                                           -L2*m3*r3*sin(q3_d)*(q2d_d + q3d_d);\n                                                                                                                                                                                                                                                                              q1d_d*((Iy3*sin(2*q2_d + 2*q3_d))/2 - (Ix3*sin(2*q2_d + 2*q3_d))/2 + (L3^2*m3*sin(2*q2_d + 2*q3_d))/2 + L1*L3*m3*sin(q2_d + q3_d) + (L2*L3*m3*sin(q3_d))/2 + (L2*L3*m3*sin(2*q2_d + q3_d))/2),                                                                                                                                                                                                                                                       L2*m3*q2d_d*r3*sin(q3_d),                                                                                                                                                                       0;];\n\nG_d = [                                                    0;\n    g*(m2*r2*cos(q2_d) + m3*r3*cos(q2_d + q3_d) + L2*m3*cos(q2_d));\n                                      g*m3*r3*cos(q2_d + q3_d);] ;\n\n\n\n\n%% Update\nTheta_s1_init = Theta_s1_init(:);\nTheta_s2_init = Theta_s2_init(:);\n%% 预处理\ntheta_hat1 = zeros(3,1);\ntheta_hat2 = zeros(3,1);\ntheta_hat3 = zeros(3,1);\ntheta_hat4 = zeros(3,1);\ntheta_hat5 = zeros(3,1);\ntheta_hat6 = zeros(3,1);\n\ntheta_hat1 (1) = Theta_Swing_F_hat (1); % fv\ntheta_hat2 (1) = Theta_Swing_F_hat (2); % fc\ntheta_hat3 (1) = Theta_Swing_F_hat (3); % D_Fn\ntheta_hat4 (1) = Theta_Swing_Q_hat (1); % 1/beta_e\ntheta_hat5 (1) = Theta_Swing_Q_hat (2); % D_Qin\ntheta_hat6 (1) = Theta_Swing_Q_hat (3); % D_Qon\n\ntheta_hat1 (2) = Theta_Boom_F_hat (1);\ntheta_hat2 (2) = Theta_Boom_F_hat (2);\ntheta_hat3 (2) = Theta_Boom_F_hat (3);\ntheta_hat4 (2) = Theta_Boom_Q_hat (1);\ntheta_hat5 (2) = Theta_Boom_Q_hat (2);\ntheta_hat6 (2) = Theta_Boom_Q_hat (3);\n\ntheta_hat1 (3) = Theta_Stick_F_hat (1);\ntheta_hat2 (3) = Theta_Stick_F_hat (2);\ntheta_hat3 (3) = Theta_Stick_F_hat (3);\ntheta_hat4 (3) = Theta_Stick_Q_hat (1);\ntheta_hat5 (3) = Theta_Stick_Q_hat (2);\ntheta_hat6 (3) = Theta_Stick_Q_hat (3);\n\n\n%% step1\nK1 = K1(:);\nK2 = K2(:);\nK3 = K3(:);\ne1 = q - qd;\ne1_dot = q_dot - qd_dot;\nqeq_dot = qd_dot - K1.*e1;\nqeq_ddot = qd_ddot - K1.*e1_dot;\ne2 = q_dot - qeq_dot;\nS_qdot = 2/pi*atan(900*q_dot);   \nSd_qdot = 2/pi*atan(900*qd_dot);   \n\nFLda1 = inv_J_h * (M_d * qeq_dot + C_d * qd_dot + G_d + theta_hat1 .* qd_dot + theta_hat2 .* Sd_qdot - theta_hat3);\nFLds1 = - inv_J_h * K2 .* e2;\nFLda2 = - inv_J_h * d1hat(:);\nFLds2 = 0;\n\nFLd = FLda1* sw_FLda1 + FLda2  + FLds1 + FLds2;\nFL = Pi.*Ai - Po.*Ao; \ne3 = FL - FLd;\n%% step2\nFLdc_dot = zeros(3,1);\n\n% QLda1 = J_h*A_Q*q_dot - B_Q*theta_hat4 - C_Q*theta_hat5 + FLdc_dot*theta_hat6 + Upsilon_Q;\nw1 = w1( : ) ;\nw2 = w2 ( : ); \nomega = w1 ./ w2 ;\n\nQLda1 = J_h*diag(A_Q) * qd_dot + diag(FLdc_dot) * theta_hat4 - diag(B_Q) * theta_hat5 - diag(C_Q) * theta_hat6 ;\nQLda2 = -d2hat( : );\nQLds1 = -K3 .* e3;     \nY_Q = -J_h * omega .* e2 * sw_Y_Q;                                    \nQLd = QLda1 * sw_QLda1 + QLda2  +  QLds1  + Y_Q; \ne2_e3 = e2./e3;\n\n\n%% ----------------------Filtering----------------------\ntau_f = 0.006 ;\ntemp_A  = [q_dot ; S_qdot ; - ones(3,1) ; B_Q ;  C_Q ; (J_h * FL + C' * q_dot - G) ] ;  % Normal Filiter var R 18*1\ntemp_B = [FL ; M * q_dot ];  % first-order Filiter var  R 6*1\n% Normal Filiter\nX1_f_next = (temp_A - X1_f( : )) / tau_f * ts + X1_f( : );\n% first-order Filiter\nX2_f_next = (temp_B - X2_f( : )) / tau_f * ts + X2_f( : ) ;\ntemp_B_dot  = (temp_B - X2_f( : )) / tau_f ;\n\nfilter_FL_dot = temp_B_dot(1 : 3);\nfilter_P_dot = temp_B_dot(4 : 6);\n\nA_f = X1_f_next(16 : 18);\nB_Q_f = X1_f_next ( 10 : 12 ) ;\nC_Q_f = X1_f_next ( 13 : 15 ) ;\nu1f_phi = filter_P_dot - A_f;\nu2f_phi = QLd - J_h * diag(A_Q) * q_dot; \n\nphi1f = reshape( X1_f_next ( 1 : 9 ) , 3 , 3 ) ;   % Arrange by column q_dot / S_qdot / - ones(3,1)\ntemp =  [ -filter_FL_dot ; B_Q_f ; C_Q_f ];\nphi2f = reshape( temp  , 3 , 3 ) ; % Arrange by column -FL_dot / B_Q / C_Q\n\n\n%%  ----------------------Theta_Updata----------------------\nF_Phi_Swing = phi1f ( 1 , : )';\nQ_Phi_Swing = phi2f ( 1 , : )';\nF_Phi_Boom= phi1f ( 2 , : )';\nQ_Phi_Boom = phi2f ( 2 , : )';\nF_Phi_Stick = phi1f ( 3 , : )';\nQ_Phi_Stick = phi2f ( 3 , : )';\n%Theta_Stick_hat = zeros(3,1);\nTheta_Swing_F_hat = Theta_Swing_F_hat( : );\nTheta_Swing_Q_hat = Theta_Swing_Q_hat( : );\nTheta_Boom_F_hat = Theta_Boom_F_hat( : );\nTheta_Boom_Q_hat = Theta_Boom_Q_hat( : );\nTheta_Stick_F_hat = Theta_Stick_F_hat( : );\nTheta_Stick_Q_hat = Theta_Stick_Q_hat( : );\nv1 = 0.1;\nv2 = 0.1;\n\n% Calculate estimation errors Epsilon\nEpsilon_1 = zeros(3, 1);\nEpsilon_2 = zeros(3, 1);\nEpsilon_1(1) = -F_Phi_Swing' * Theta_Swing_F_hat - u1f_phi(1);   % Swing\nEpsilon_1(2) = -F_Phi_Boom' * Theta_Boom_F_hat - u1f_phi(2);     % Boom\nEpsilon_1(3) = -F_Phi_Stick' * Theta_Stick_F_hat - u1f_phi(3);   % Stick\n\nEpsilon_2(1) = -Q_Phi_Swing' * Theta_Swing_Q_hat - u2f_phi(1);   % Swing\nEpsilon_2(2) = -Q_Phi_Boom' * Theta_Boom_Q_hat - u2f_phi(2);     % Boom\nEpsilon_2(3) = -Q_Phi_Stick' * Theta_Stick_Q_hat - u2f_phi(3);   % Stick\n\n% Calculate xi\nxi_1 = zeros(3, 1);\nxi_2 = zeros(3, 1);\nxi_1(1) = 1 / (1 + v1 * F_Phi_Swing' * Gamma_1_Swing * F_Phi_Swing);  % Swing\nxi_1(2) = 1 / (1 + v1 * F_Phi_Boom' * Gamma_1_Boom * F_Phi_Boom);     % Boom\nxi_1(3) = 1 / (1 + v1 * F_Phi_Stick' * Gamma_1 * F_Phi_Stick);        % Stick\n\nxi_2(1) = 1 / (1 + v2 * Q_Phi_Swing' * Gamma_2_Swing * Q_Phi_Swing);  % Swing\nxi_2(2) = 1 / (1 + v2 * Q_Phi_Boom' * Gamma_2_Boom * Q_Phi_Boom);     % Boom\nxi_2(3) = 1 / (1 + v2 * Q_Phi_Stick' * Gamma_2 * Q_Phi_Stick);        % Stick\n\n% Since tau vectors might have different dimensions, store them separately\ntau_1_Swing = xi_1(1) * F_Phi_Swing * Epsilon_1(1);  % Swing\ntau_1_Boom = xi_1(2) * F_Phi_Boom * Epsilon_1(2);    % Boom\ntau_1_Stick = xi_1(3) * F_Phi_Stick * Epsilon_1(3);  % Stick\n\ntau_2_Swing = xi_2(1) * Q_Phi_Swing * Epsilon_2(1);  % Swing\ntau_2_Boom = xi_2(2) * Q_Phi_Boom * Epsilon_2(2);    % Boom\ntau_2_Stick = xi_2(3) * Q_Phi_Stick * Epsilon_2(3);  % Stick\n\n% Calculate derivatives of Theta_hat\nTheta_Swing_F_hat_dot = Gamma_1_Swing * tau_1_Swing;  % Swing\nTheta_Boom_F_hat_dot = Gamma_1_Boom * tau_1_Boom;     % Boom\nTheta_Stick_F_hat_dot = Gamma_1 * tau_1_Stick;        % Stick\n\nTheta_Swing_Q_hat_dot = Gamma_2_Swing * tau_2_Swing;  % Swing\nTheta_Boom_Q_hat_dot = Gamma_2_Boom * tau_2_Boom;     % Boom\nTheta_Stick_Q_hat_dot = Gamma_2 * tau_2_Stick;        % Stick\n\n% Calculate Theta_hat for next time step\nTheta_Swing_F_hat_next = Theta_Swing_F_hat_dot * ts + Theta_Swing_F_hat;  % Swing\nTheta_Boom_F_hat_next = Theta_Boom_F_hat_dot * ts + Theta_Boom_F_hat;     % Boom\nTheta_Stick_F_hat_next = Theta_Stick_F_hat_dot * ts + Theta_Stick_F_hat;  % Stick\n\nTheta_Swing_Q_hat_next = Theta_Swing_Q_hat_dot * ts + Theta_Swing_Q_hat;  % Swing\nTheta_Boom_Q_hat_next = Theta_Boom_Q_hat_dot * ts + Theta_Boom_Q_hat;     % Boom\nTheta_Stick_Q_hat_next = Theta_Stick_Q_hat_dot * ts + Theta_Stick_Q_hat;  % Stick\n\n% Parameter limits\nTheta_Swing_Max = [2000, 20000, 200, 1/(2e8), 1e-5, 1e-5];  % fv fc D_Fn D_Qin D_Qon 1/beta\nTheta_Swing_Min = [10,      10,     -200, 1/(1.25e9), -1e-5, -1e-5];\nTheta_Boom_Max = [2000, 20000, 200, 1/(2e8), 1e-5, 1e-5];  % fv fc D_Fn D_Qin D_Qon 1/beta\nTheta_Boom_Min = [10,      10,     -200, 1/(1.25e9), -1e-5, -1e-5];\nTheta_Stick_Max = [2000, 20000, 200, 1/(2e8), 1e-5, 1e-5];  % fv fc D_Fn D_Qin D_Qon 1/beta\nTheta_Stick_Min = [10,      10,     -200, 1/(1.25e9), -1e-5, -1e-5];\n\nTheta_Swing_Max = [2000, 20000, 200, 1/(2e8), 1e-1, 1e-1];  % fv fc D_Fn D_Qin D_Qon 1/beta\nTheta_Swing_Min = [10,      10,     -200, 1/(1.25e9), -1e-1, -1e-1];\n\nTheta_Boom_Max = [2000, 20000, 200, 1/(2e8), 1e-1, 1e-1];  % fv fc D_Fn D_Qin D_Qon 1/beta\nTheta_Boom_Min = [10,      10,     -200, 1/(1.25e9), -1e-1, -1e-1];\n\nTheta_Stick_Max = [2000, 20000, 200, 1/(2e8), 1e-1, 1e-1];  % fv fc D_Fn D_Qin D_Qon 1/beta\nTheta_Stick_Min = [10,      10,     -200, 1/(1.25e9), -1e-1, -1e-1];\n\n% Apply parameter limits\nfor idx = 1:3\n    %Swing\n    Theta_Swing_F_hat_next(idx) = min(max(Theta_Swing_F_hat_next(idx), Theta_Swing_Min(idx)), Theta_Swing_Max(idx));\n    Theta_Swing_Q_hat_next(idx) = min(max(Theta_Swing_Q_hat_next(idx), Theta_Swing_Min(idx + 3)), Theta_Swing_Max(idx + 3));\n    \n    %Boom\n    Theta_Boom_F_hat_next(idx) = min(max(Theta_Boom_F_hat_next(idx), Theta_Boom_Min(idx)), Theta_Boom_Max(idx));\n    Theta_Boom_Q_hat_next(idx) = min(max(Theta_Boom_Q_hat_next(idx), Theta_Boom_Min(idx + 3)), Theta_Boom_Max(idx + 3));\n    \n    %Stick\n    Theta_Stick_F_hat_next(idx) = min(max(Theta_Stick_F_hat_next(idx), Theta_Stick_Min(idx)), Theta_Stick_Max(idx));\n    Theta_Stick_Q_hat_next(idx) = min(max(Theta_Stick_Q_hat_next(idx), Theta_Stick_Min(idx + 3)), Theta_Stick_Max(idx + 3));\nend\n\n\nif  Use_Preset_Theta == 1\n    Theta_Swing_F_hat_next = [Theta_s1_init(1);Theta_s1_init(4);Theta_s1_init(7)];\n    Theta_Boom_F_hat_next = [Theta_s1_init(2);Theta_s1_init(5);Theta_s1_init(8)];\n    Theta_Stick_F_hat_next = [Theta_s1_init(3);Theta_s1_init(6);Theta_s1_init(9)];\n    Theta_Swing_Q_hat_next = [Theta_s2_init(1);Theta_s2_init(4);Theta_s2_init(7)];\n    Theta_Boom_Q_hat_next = [Theta_s2_init(2);Theta_s2_init(5);Theta_s2_init(8)];\n    Theta_Stick_Q_hat_next = [Theta_s2_init(3);Theta_s2_init(6);Theta_s2_init(9)];\nend\n\n\nif  Stop_Theta_Update == 1\n    Theta_Swing_F_hat_next = Theta_Swing_F_hat;\n    Theta_Boom_F_hat_next = Theta_Boom_F_hat;\n    Theta_Stick_F_hat_next = Theta_Stick_F_hat;\n    Theta_Swing_Q_hat_next = Theta_Swing_Q_hat;\n    Theta_Boom_Q_hat_next = Theta_Boom_Q_hat;\n    Theta_Stick_Q_hat_next = Theta_Stick_Q_hat;\nend\n%% ----------------------Gamma_Update----------------------\n% Update rates\nalpha_1 = 0.2;\nalpha_2 = 0.2;\n\n% Calculate Gamma derivatives\nGamma_1_Swing_dot = alpha_1 * Gamma_1_Swing - xi_1(1) * Gamma_1_Swing * F_Phi_Swing' * F_Phi_Swing * Gamma_1_Swing;\nGamma_1_Boom_dot = alpha_1 * Gamma_1_Boom - xi_1(2) * Gamma_1_Boom * F_Phi_Boom' * F_Phi_Boom * Gamma_1_Boom;\nGamma_1_dot = alpha_1 * Gamma_1 - xi_1(3) * Gamma_1 * F_Phi_Stick' * F_Phi_Stick * Gamma_1;\n\nGamma_2_Swing_dot = alpha_2 * Gamma_2_Swing - xi_2(1) * Gamma_2_Swing * Q_Phi_Swing' * Q_Phi_Swing * Gamma_2_Swing;\nGamma_2_Boom_dot = alpha_2 * Gamma_2_Boom - xi_2(2) * Gamma_2_Boom * Q_Phi_Boom' * Q_Phi_Boom * Gamma_2_Boom;\nGamma_2_dot = alpha_2 * Gamma_2 - xi_2(3) * Gamma_2 * Q_Phi_Stick' * Q_Phi_Stick * Gamma_2;\n\n% Update Gamma matrices\nGamma_1_Swing_next = Gamma_1_Swing_dot * ts + Gamma_1_Swing;\nGamma_1_Boom_next = Gamma_1_Boom_dot * ts + Gamma_1_Boom;\nGamma_1_next = Gamma_1_dot * ts + Gamma_1;\n\nGamma_2_Swing_next = Gamma_2_Swing_dot * ts + Gamma_2_Swing;\nGamma_2_Boom_next = Gamma_2_Boom_dot * ts + Gamma_2_Boom;\nGamma_2_next = Gamma_2_dot * ts + Gamma_2;\n\n% Gamma limits\nGamma_1_Max = [1000, 1000, 1000];\nGamma_1_Min = -Gamma_1_Max;\nGamma_2_Max = [1e-1, 1e-3, 1e-3];\nGamma_2_Min = -Gamma_2_Max;\n\n% Apply Gamma limits\nfor idx = 1:3\n    % Swing\n    Gamma_1_Swing_next  = min(max(Gamma_1_Swing_next , Gamma_1_Min(idx)), Gamma_1_Max(idx));\n    Gamma_2_Swing_next  = min(max(Gamma_2_Swing_next , Gamma_2_Min(idx)), Gamma_2_Max(idx));\n    \n    % Boom\n    Gamma_1_Boom_next  = min(max(Gamma_1_Boom_next , Gamma_1_Min(idx)), Gamma_1_Max(idx));\n    Gamma_2_Boom_next  = min(max(Gamma_2_Boom_next , Gamma_2_Min(idx)), Gamma_2_Max(idx));\n    \n    % Stick\n    Gamma_1_next = min(max(Gamma_1_next , Gamma_1_Min(idx)), Gamma_1_Max(idx));\n    Gamma_2_next  = min(max(Gamma_2_next , Gamma_2_Min(idx)), Gamma_2_Max(idx));\nend\n\n\n%% ----------------------dihat_Updata----------------------\n\nd1hat_dot = diag(gamma_d1) * e2;\nd2hat_dot = diag(gamma_d2) * e3;\nd1hat_next = d1hat_dot * ts + d1hat(:);\nd2hat_next = d2hat_dot * ts + d2hat(:);\nd1max = ones(3 ,1) * 1e2;\nd2max = ones(3 ,1) * 5e-4;\nd1min = -d1max;\nd2min = -d2max;\nfor idx = 1 : 3\n   if d1hat_next(idx) > d1max(idx)\n       d1hat_next(idx) = d1max(idx);\n   end\n    if d1hat_next(idx) < d1min(idx)\n       d1hat_next(idx) = d1min(idx);\n   end\n\n   if d2hat_next(idx) > d2max(idx)\n       d2hat_next(idx) = d2max(idx);\n    end\n    if d2hat_next(idx) < d2min(idx)\n       d2hat_next(idx) = d2min(idx);\n    end\nend\nif sw_d1hat == 0\n    d1hat_next = zeros(3,1);\nend\nif sw_d2hat == 0\n    d2hat_next = zeros(3,1);\nend\n\n%%\n% Q to U\nPr = 0;                                     \nkq1 = 1.069e-9;                         \t\nkq2 = 1.069e-9;                           \t\nk = 10;                                    \t\n\nif QLd > 0 % forword\n    Delta_p1 = Ps - Pi;\n    Delta_p2 = Po - Pr;\nelse % backspacings\n    Delta_p1 = Pi - Pr;\n    Delta_p2 = Ps - Po;\nend\n\nXv = QLd ./ (Ai./Vi.*kq1.*sqrt(Delta_p1) + Ao./Vo.*kq2.*sqrt(Delta_p2));\nU = 1./k .* Xv;          \n\nUmax = 5;\nfor idx = 1 : 3\n    if U(idx) > Umax\n        U(idx) = Umax;\n    end\n    if U(idx) < -Umax\n        U(idx) = -Umax;\n    end\nend\n\n\n\n\n%%  ————————detect——————————\n% F组：每行是一个动作的数据列\nF_Swing = [FLd(1); FLda1(1); FLds1(1); FLda2(1)];\nF_Boom  = [FLd(2); FLda1(2); FLds1(2); FLda2(2)];\nF_Stick = [FLd(3); FLda1(3); FLds1(3); FLda2(3)];\n\n% Q组\nQ_Swing = [QLd(1); QLda1(1); QLds1(1); QLda2(1)];\nQ_Boom  = [QLd(2); QLda1(2); QLds1(2); QLda2(2)];\nQ_Stick = [QLd(3); QLda1(3); QLds1(3); QLda2(3)];" ("Base Controller")("q1"=w370, "q2"=w332, "q3"=w331, "alpha1"=w368, "alpha2"=w367, "alpha3"=w364, "pi1"=w362, "pi2"=w353, "pi3"=w354, "po1"=w355, "po2"=w356, "po3"=w357, "ts"=w344, "Ps"=w352, "Desired_Swing"=w335, "Desired_Boom"=w334, "Desired_Stick"=w333, "K1"="K1", "K2"="K2", "K3"=w318, "q_dot_f"=w272, "q_f"=w273, "Desired_q_Swing"=w326, "Desired_q_Boom"=w327, "Desired_q_Stick"=w328, "sw_QLda1"="sw_QLda1", "sw_FLda1"="sw_FLda1", "Theta_s1_init"="Theta_s1_init", "Theta_s2_init"=w311, "gamma_d1"="gamma_d1", "gamma_d2"=w321, "d1hat"=w317, "d2hat"=w315, "sw_d1hat"="sw_d1hat", "sw_d2hat"="sw_d2hat", "X1_f"=w310, "X2_f"=w309, "Gamma_1"=w260, "Theta_Stick_F_hat"=w304, "Gamma_2"=w258, "Theta_Stick_Q_hat"=w302, "Gamma_1_Swing"=w268, "Gamma_1_Boom"=w264, "Gamma_2_Swing"=w266, "Gamma_2_Boom"=w262, "Theta_Swing_F_hat"=w300, "Theta_Swing_Q_hat"=w298, "Theta_Boom_Q_hat"=w295, "Theta_Boom_F_hat"=w296, "w1"="w1", "w2"="w2", "sw_Y_Q"="sw_Y_Q", "Stop_Theta_Update"="Stop\nTheta_Update", "Use_Preset_Theta"="Use\nPreset_Theta") -> ("q_dot_f_next"=w269:dbl[], "q_f_next"=w270:dbl[], "U"=w340:dbl[], "d1hat_next"=w316:dbl[], "d2hat_next"=w314:dbl[], "X2_f_next"=w308:dbl[], "X1_f_next"=w307:dbl[], "Gamma_1_next"=w259:dbl, "Theta_Stick_F_hat_next"=w248:dbl[], "Theta_Stick_Q_hat_next"=w245:dbl[], "Gamma_2_next"=w257:dbl, "Gamma_1_Swing_next"=w267:dbl, "Gamma_2_Swing_next"=w265:dbl, "Gamma_1_Boom_next"=w263:dbl, "Gamma_2_Boom_next"=w261:dbl, "Theta_Swing_F_hat_next"=w299:dbl[], "Theta_Swing_Q_hat_next"=w297:dbl[], "Theta_Boom_Q_hat_next"=w241:dbl[], "Theta_Boom_F_hat_next"=w242:dbl[], "Epsilon_1"=w291:cdb[], "Epsilon_2"=w289:cdb[], "e2"=→"e2":dbl[], "e3"=→"e3":dbl[], "F_Swing"=w288:cdb[], "F_Boom"=w279:cdb[], "F_Stick"=w278:cdb[], "Q_Swing"=w280:cdb[], "Q_Stick"=w282:cdb[], "Q_Boom"=w281:cdb[], "e2_e3"=→"e2_e3":dbl[])  [unwired: 1 in, 9 out]
    "ARC_U" <- w340
    "Theta_Stick_F_hat_next" <- w248
    "Theta_Stick_Q_hat_next" <- w245
    "Theta_Swing_F_hat_next" <- w299
    "Theta_Swing_Q_hat_next" <- w297
    "Theta_Boom_F_hat_next" <- w242
    "Theta_Boom_Q_hat_next" <- w241
    n193 = Array To Cluster(array=w282) -> (cluster=→"Q_Stick":T13)
    n194 = Array To Cluster(array=w281) -> (cluster=→"Q_Boom":T14)
    n195 = Array To Cluster(array=w280) -> (cluster=→"Q_Swing":T15)
    n196 = Array To Cluster(array=w278) -> (cluster=→"F_Stick":T16)
    n197 = Array To Cluster(array=w279) -> (cluster=→"F_Boom":T17)
    n198 = Array To Cluster(array=w288) -> (cluster=→"F_Swing":T18)
    n199 = feedback-in #3(w269) -> ()
    n200 = feedback-in #4(w270) -> ()
    n201 = feedback-in #5(w242) -> ()
    n202 = feedback-in #6(w241) -> ()
    n203 = feedback-in #7(w297) -> ()
    n204 = feedback-in #8(w245) -> ()
    n205 = feedback-in #9(w267) -> ()
    n206 = feedback-in #10(w265) -> ()
    n207 = feedback-in #11(w263) -> ()
    n208 = feedback-in #12(w261) -> ()
    n209 = feedback-in #13(w259) -> ()
    n210 = feedback-in #14(w257) -> ()
    n211 = feedback-in #15(w299) -> ()
    n212 = feedback-in #16(w248) -> ()
    n213 = feedback-in #17(w316) -> ()
    n214 = feedback-in #18(w314) -> ()
    n215 = feedback-in #19(w307) -> ()
    n216 = feedback-in #20(w308) -> ()
    n217 = Array Size(array=w340) -> ()  [unwired: 1 out]
    n218 = Index Array(array=w340, index=1) -> (element=w336:dbl)
    n219 = Index Array(array=w340, index=0) -> (element=w341:dbl)
    n220 = Index Array(array=w340, index=2) -> (element=w337:dbl)
    n221 = shared-variable ".\\sharedV.lvlib\\ARC_U_Swing"(w341) -> ()  [unwired: 1 in, 1 out]
    n222 = Array To Cluster(array=w291) -> (cluster=→"Esti_e1":T19)
    n223 = Array To Cluster(array=w289) -> (cluster=→"Esti_e2":T20)
    n224 = expression code="(x/pi)*180.0" ("弧度转换至角度")(w270) -> (w329:dbl[])
    n225 = expression code="(x/pi)*180.0" ("弧度转换至角度")(w269) -> (w330:dbl[])
    n226 = shared-variable ".\\sharedV.lvlib\\q_dot_f"(w329) -> ()  [unwired: 1 in, 1 out]
    n227 = shared-variable ".\\sharedV.lvlib\\ARC_U_Boom"(w336) -> ()  [unwired: 1 in, 1 out]
    n228 = shared-variable ".\\sharedV.lvlib\\ARC_U_Stick"(w337) -> ()  [unwired: 1 in, 1 out]
    n229 = shared-variable ".\\sharedV.lvlib\\q_f"(w330) -> ()  [unwired: 1 in, 1 out]
    n230 = Array To Cluster(array=w245) -> (cluster=→"Theta_Stick_Q_hat_next":T21)
    n231 = Array To Cluster(array=w248) -> (cluster=→"Theta_Stick_F_hat_next":T7)
    n232 = Array To Cluster(array=w241) -> (cluster=→"Theta_Boom_Q_hat_next":T22)
    n233 = Array To Cluster(array=w242) -> (cluster=→"Theta_Boom_F_hat_next":T23)
    n234 = node-c288() -> ()  [unwired: 1 in, 1 out]
  }
  n235 = node-c288(w19) -> ()  [unwired: 1 out]
